vi "FPGA_Host_RealTime_Data_Viewer.vi"(3 "length":i32, 4 "Array":dbl[][](array[numeric]), 5 "Display Cluster":T1) -> ()   [LabVIEW 2023]
uses:
  TypeDefs/Display.ctl
  <vilib>/Analysis/baseanly.llb/Mean (DBL).vi
  User_Vi/Settings.vi
  <vilib>/Analysis/NI_AALBase.lvlib
panel:
  out "Current 3":bool=TRUE
  out "Forward Current3":dbl[][](array[numeric])
  out "Reverse Current3":dbl[][](array[numeric])
  out "Raster Current 3":dbl[][](array[numeric])
  out "Reverse Current2":dbl[][](array[numeric])
  out "Forward Current2":dbl[][](array[numeric])
  out "Current 2":bool=TRUE
  out "Raster Current 2":dbl[][](array[numeric])
  out "Current 1":bool=TRUE
  out "Reverse Current1":dbl[][](array[numeric])
  out "Forward Current1":dbl[][](array[numeric])
  out "Raster Current1":dbl[][](array[numeric])
  out "Raster Topo":dbl[][](array[numeric])
  out "Hop Current3":dbl[][](array[numeric])
  in  "Hop C3":bool=TRUE
  out "Hop Current2":dbl[][](array[numeric])
  in  "Hop C2":bool=TRUE
  out "Hop Current1":dbl[][](array[numeric])
  in  "Hop C1":bool=TRUE
  in  "Hop Top":bool=TRUE
  out "Hop Topography":dbl[][](array[numeric])
  out "Topology":bool=TRUE
  out "Reverse Topo":dbl[][](array[numeric])
  out "Forward Topo":dbl[][](array[numeric])
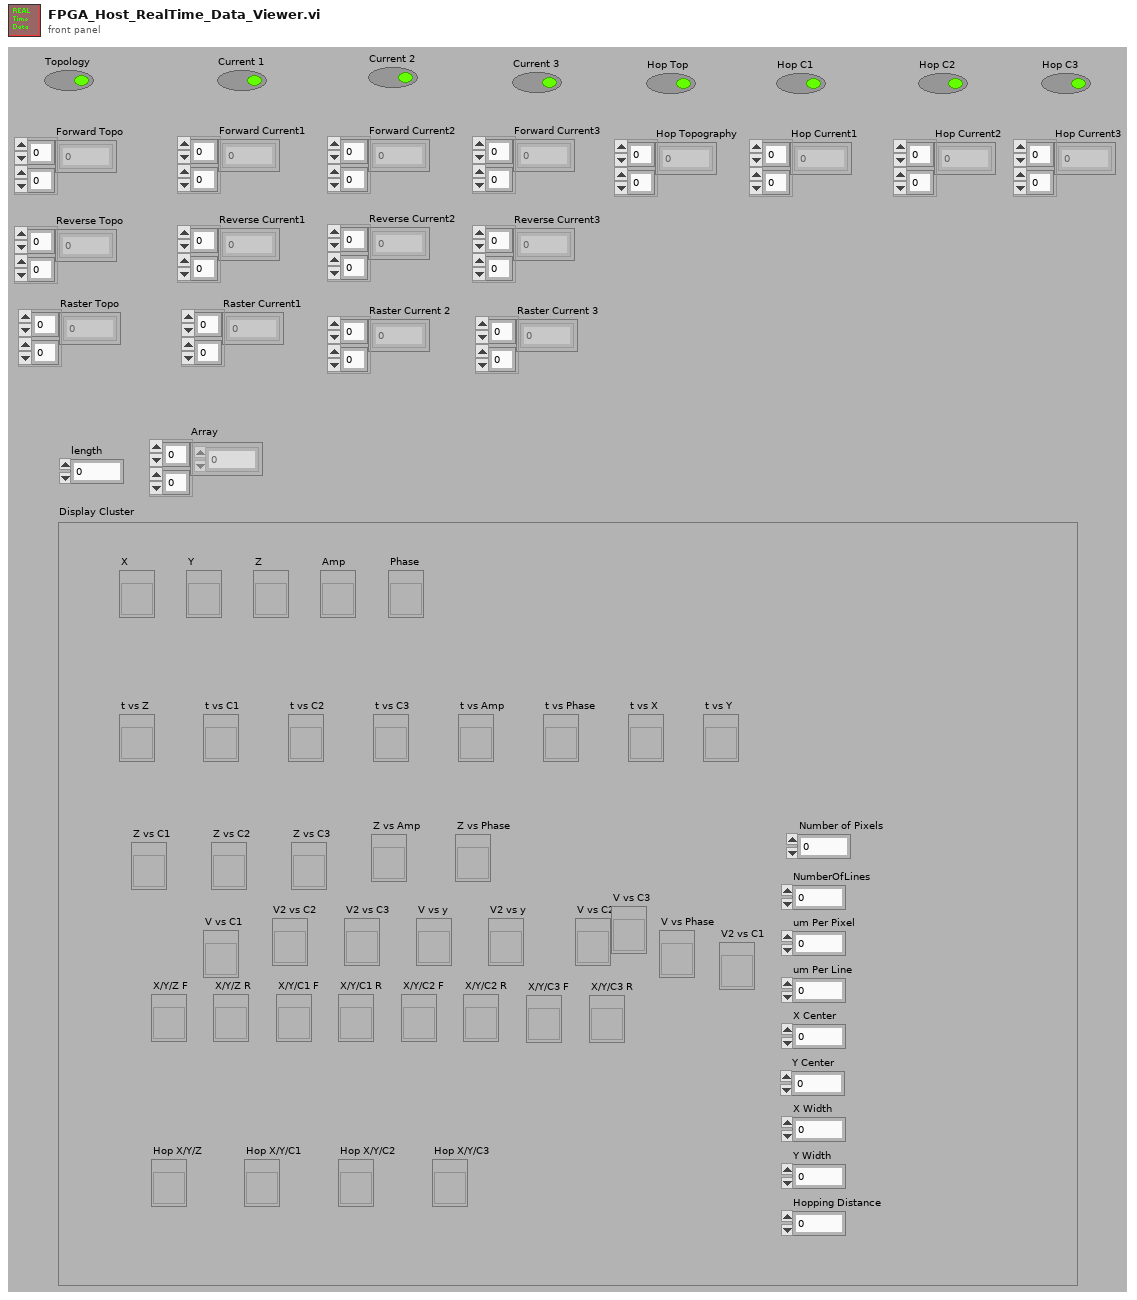
[diagram p1: front panel]
types:
  T1 = typedef "Display.ctl" = cluster{"X":refnum<vi>, "Y":refnum<vi>, "Z":refnum<vi>, "Amp":refnum<vi>, "Phase":refnum<vi>, "t vs Z":refnum<vi>, "t vs C1":refnum<vi>, "t vs C2":refnum<vi>, "t vs C3":refnum<vi>, "t vs Amp":refnum<vi>, "t vs Phase":refnum<vi>, "t vs X":refnum<vi>, "t vs Y":refnum<vi>, "Z vs C1":refnum<vi>, "Z vs C2":refnum<vi>, "Z vs C3":refnum<vi>, "V vs C1":refnum<vi>, "V vs C2":refnum<vi>, "V vs C3":refnum<vi>, "X/Y/Z F":refnum<vi>, "X/Y/Z R":refnum<vi>, "X/Y/C1 F":refnum<vi>, "X/Y/C1 R":refnum<vi>, "X/Y/C2 F":refnum<vi>, "X/Y/C2 R":refnum<vi>, "X/Y/C3 F":refnum<vi>, "X/Y/C3 R":refnum<vi>, "NumberOfLines":u16, "um Per Pixel":dbl, "um Per Line":dbl, "X Center":dbl, "Hop X/Y/Z":refnum<vi>, "Hop X/Y/C1":refnum<vi>, "Hop X/Y/C2":refnum<vi>, "Hop X/Y/C3":refnum<vi>, "X Width":dbl, "Y Width":dbl, "Hopping Distance":dbl, "V2 vs C1":refnum<vi>, "V vs Phase":refnum<vi>, "Y Center":dbl, "Number of Pixels":dbl, "V2 vs C2":refnum<vi>, "V2 vs C3":refnum<vi>, "V vs y":refnum<vi>, "V2 vs y":refnum<vi>, "Z vs Amp":refnum<vi>, "Z vs Phase":refnum<vi>}
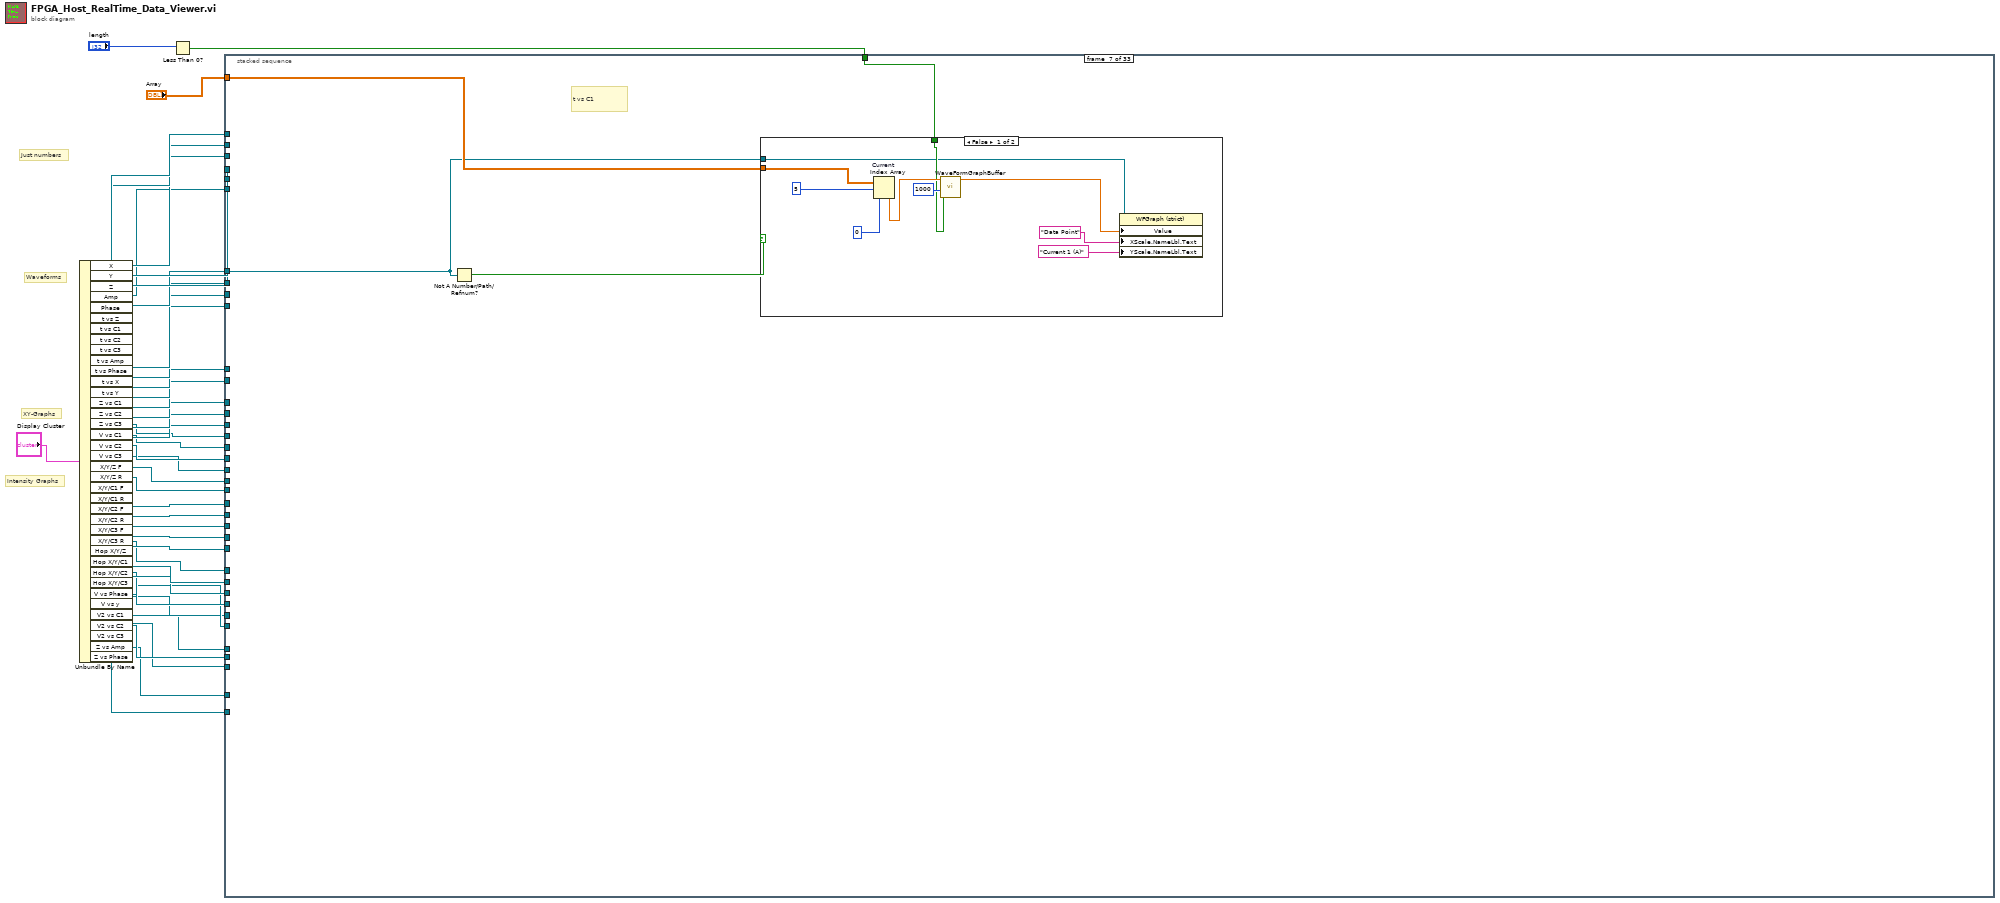
[diagram p0: block diagram]
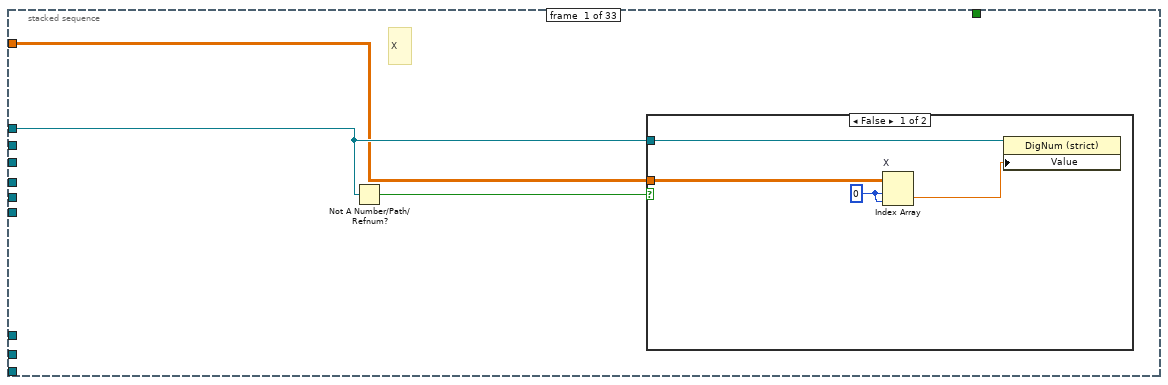
[diagram p2: hidden frame]
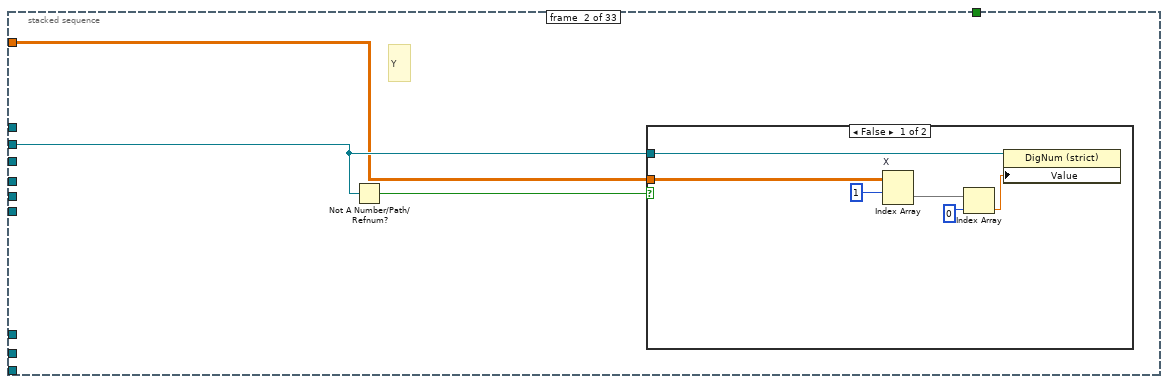
[diagram p4: hidden frame]
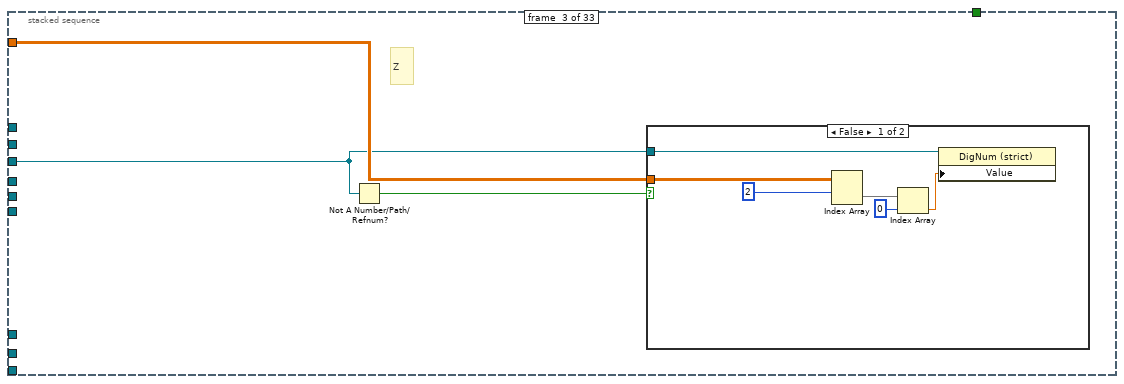
[diagram p6: hidden frame]
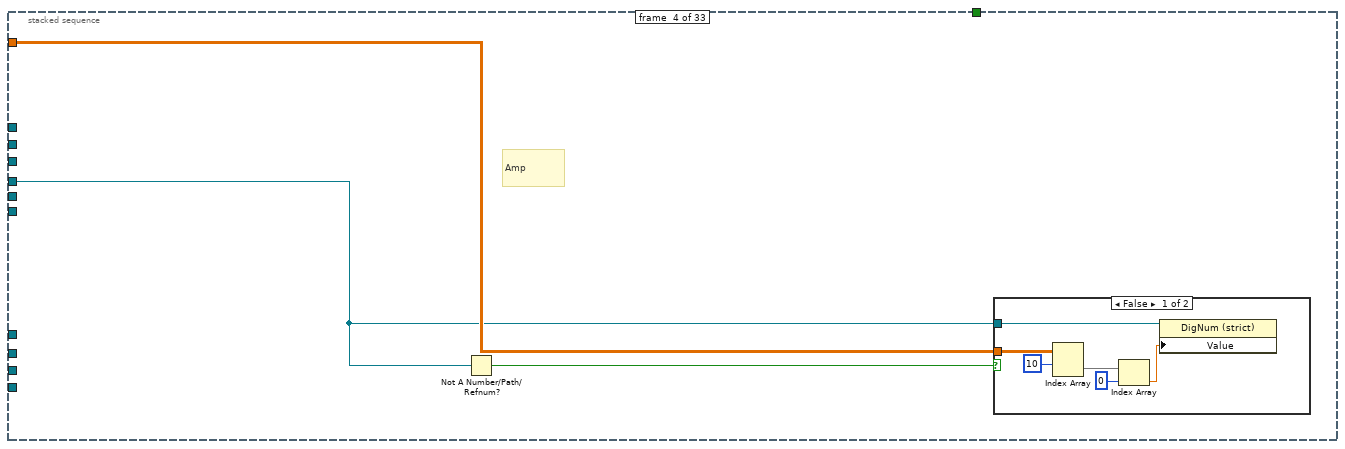
[diagram p8: hidden frame]
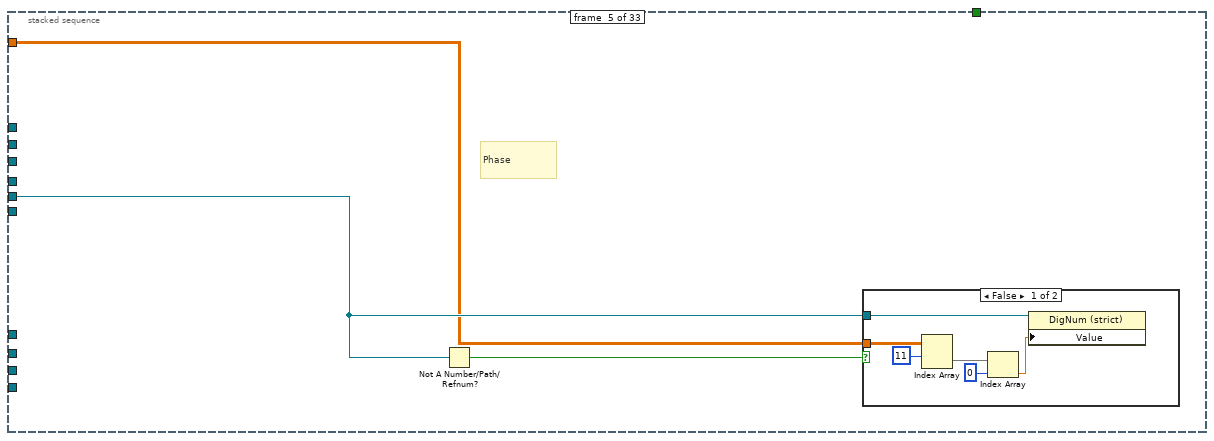
[diagram p10: hidden frame]
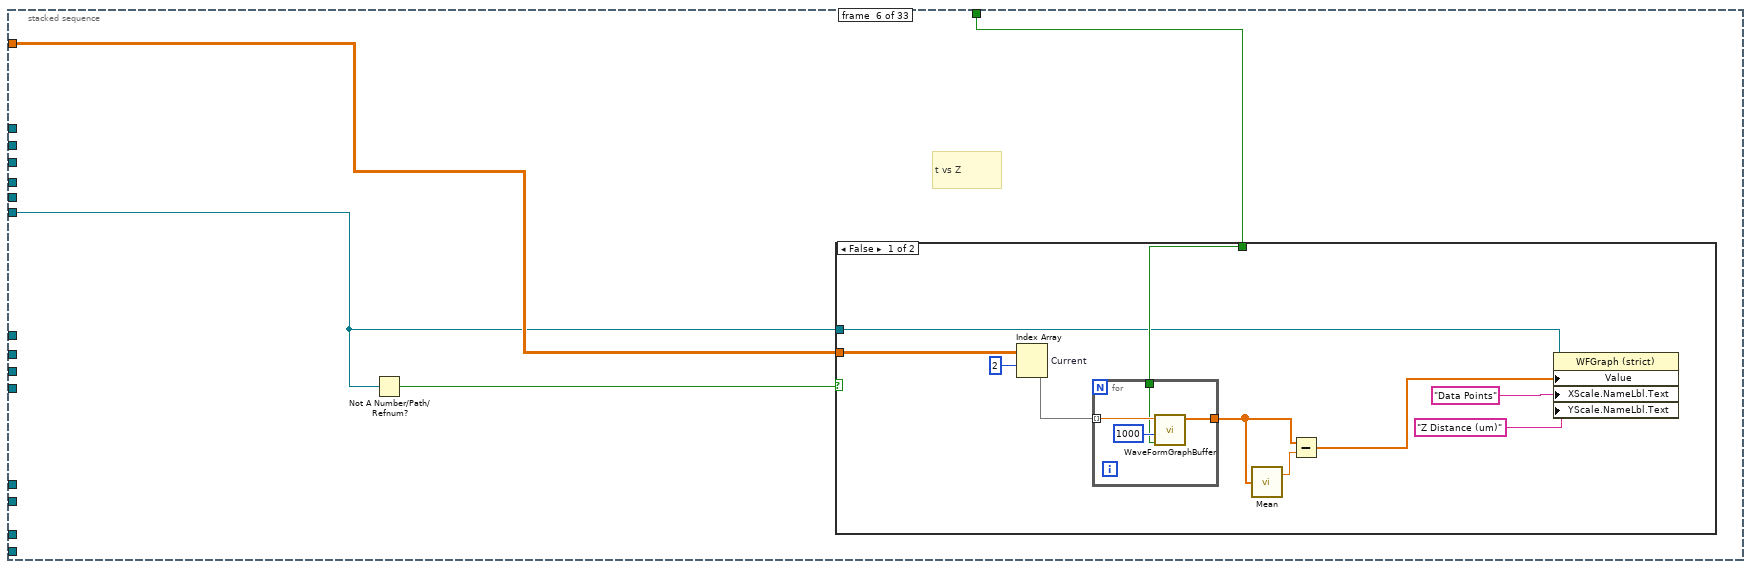
[diagram p12: hidden frame]
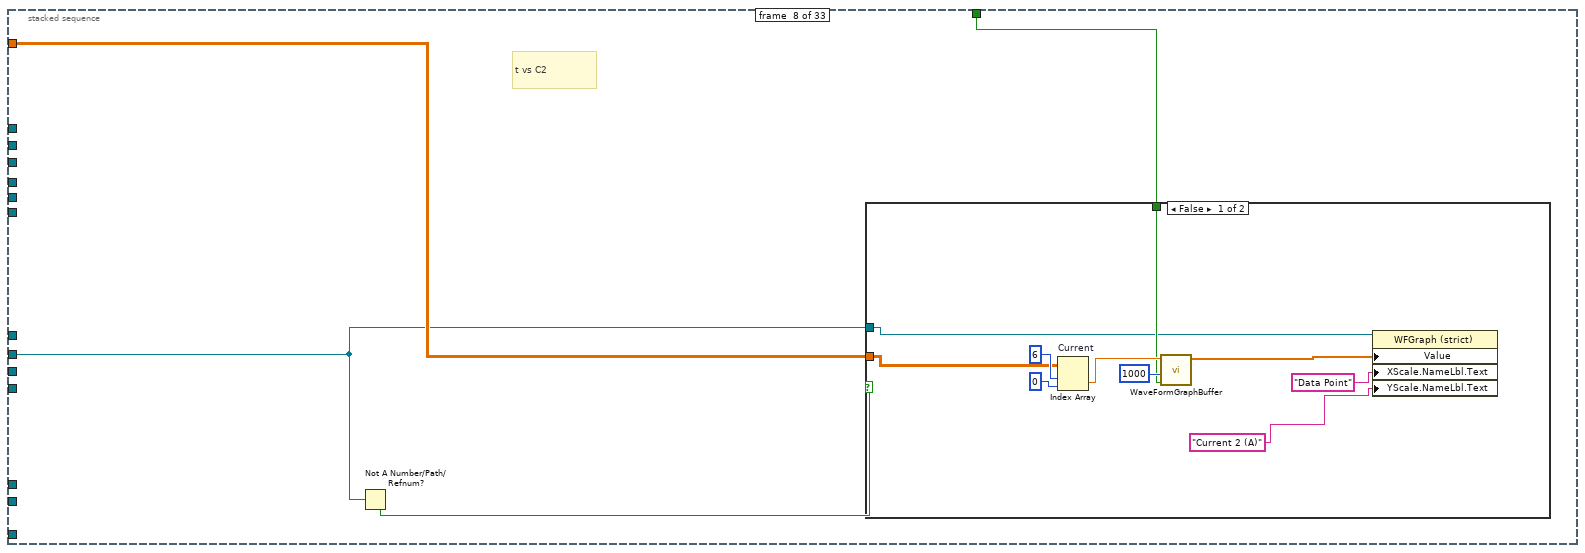
[diagram p15: hidden frame]
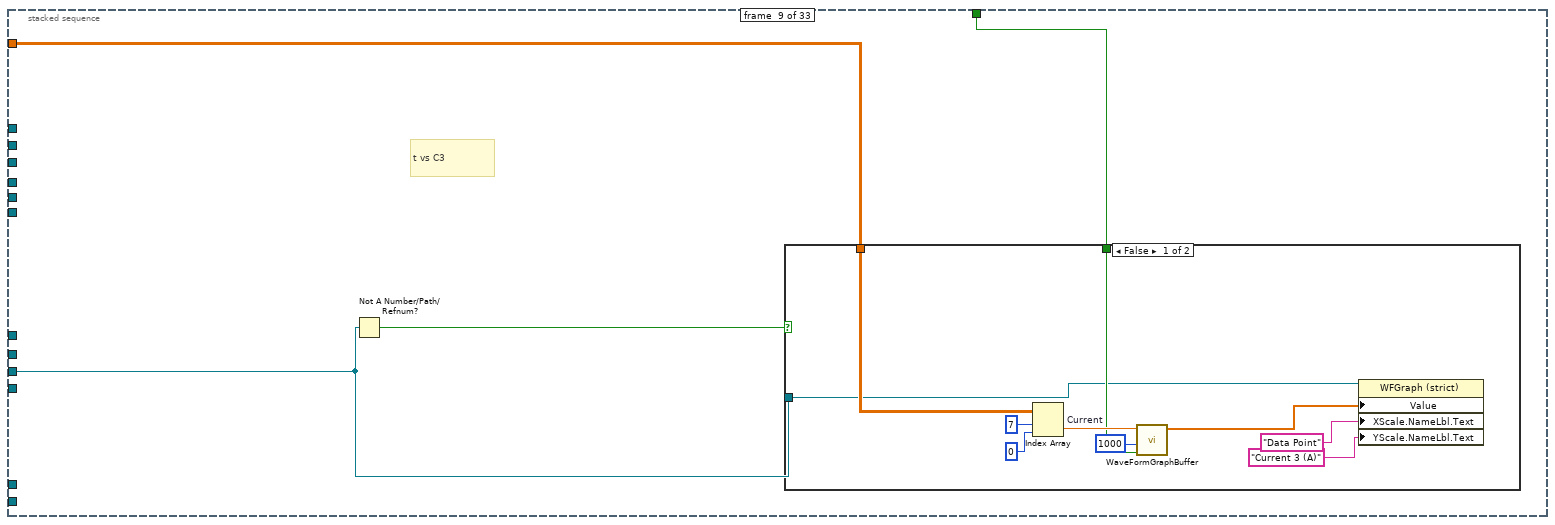
[diagram p17: hidden frame]
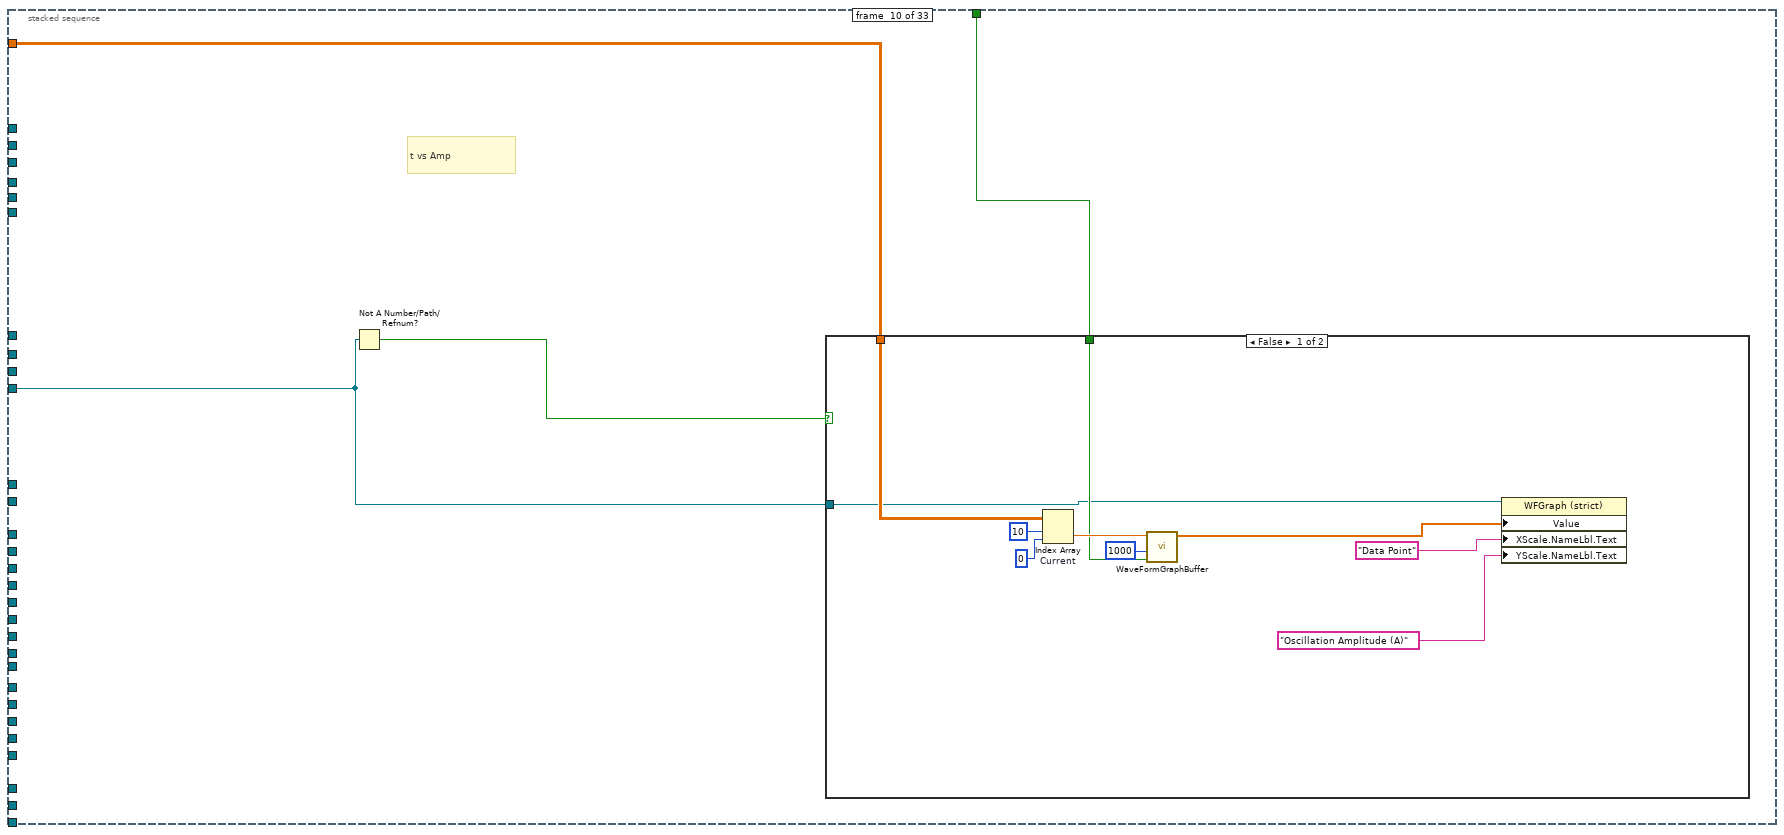
[diagram p19: hidden frame]
diagram:
  # "Intensity Graphs"
  # "XY-Graphs"
  # "Waveforms"
  # "Just numbers"
  n1 = Unbundle By Name("Display Cluster") -> ("X"=w38:refnum<vi>, "Y"=w37:refnum<vi>, "Z"=w36:refnum<vi>, "Amp"=w35:refnum<vi>, "Phase"=w34:refnum<vi>, "t vs Z"=w33:refnum<vi>, "t vs C1"=w32:refnum<vi>, "t vs C2"=w31:refnum<vi>, "t vs C3"=w30:refnum<vi>, "t vs Amp"=w29:refnum<vi>, "t vs Phase"=w28:refnum<vi>, "t vs X"=w27:refnum<vi>, "t vs Y"=w26:refnum<vi>, "Z vs C1"=w25:refnum<vi>, "Z vs C2"=w24:refnum<vi>, "Z vs C3"=w23:refnum<vi>, "V vs C1"=w22:refnum<vi>, "V vs C2"=w21:refnum<vi>, "V vs C3"=w20:refnum<vi>, "X/Y/Z F"=w19:refnum<vi>, "X/Y/Z R"=w18:refnum<vi>, "X/Y/C1 F"=w17:refnum<vi>, "X/Y/C1 R"=w16:refnum<vi>, "X/Y/C2 F"=w15:refnum<vi>, "X/Y/C2 R"=w14:refnum<vi>, "X/Y/C3 F"=w13:refnum<vi>, "X/Y/C3 R"=w6:refnum<vi>, "Hop X/Y/Z"=w12:refnum<vi>, "Hop X/Y/C1"=w11:refnum<vi>, "Hop X/Y/C2"=w10:refnum<vi>, "Hop X/Y/C3"=w7:refnum<vi>, "V vs Phase"=w8:refnum<vi>, "V2 vs C1"=w4:refnum<vi>, "V2 vs C2"=w5:refnum<vi>, "V2 vs C3"=w3:refnum<vi>, "Z vs Amp"=w2:refnum<vi>, "Z vs Phase"=w1:refnum<vi>)  [unwired: 1 out]
  n2 = Less Than 0?(x="length") -> (x < 0?=w40:bool)
  n3 = stacked-sequence {
    tunnel: w38 -> [w43 _ _ _ _ _ _ _ _ _ _ _ _ _ _ _ _ _ _ _ _ _ _ _ _ _ _ _ _ _ _ _ _]
    tunnel: w37 -> [_ w50 _ _ _ _ _ _ _ _ _ _ _ _ _ _ _ _ _ _ _ _ _ _ _ _ _ _ _ _ _ _ _]
    tunnel: w36 -> [_ _ w58 _ _ _ _ _ _ _ _ _ _ _ _ _ _ _ _ _ _ _ _ _ _ _ _ _ _ _ _ _ _]
    tunnel: w32 -> [_ _ _ _ _ _ w103 _ _ _ _ _ _ _ _ _ _ _ _ _ _ _ _ _ _ _ _ _ _ _ _ _ _]
    tunnel: w31 -> [_ _ _ _ _ _ _ w117 _ _ _ _ _ _ _ _ _ _ _ _ _ _ _ _ _ _ _ _ _ _ _ _ _]
    tunnel: w30 -> [_ _ _ _ _ _ _ _ w131 _ _ _ _ _ _ _ _ _ _ _ _ _ _ _ _ _ _ _ _ _ _ _ _]
    tunnel: w29 -> [_ _ _ _ _ _ _ _ _ w145 _ _ _ _ _ _ _ _ _ _ _ _ _ _ _ _ _ _ _ _ _ _ _]
    tunnel: w28 -> [_ _ _ _ _ _ _ _ _ _ w159 _ _ _ _ _ _ _ _ _ _ _ _ _ _ _ _ _ _ _ _ _ _]
    tunnel: w25 -> [_ _ _ _ _ _ _ _ _ _ _ _ _ w203 _ _ _ _ _ _ _ _ _ _ _ _ _ _ _ _ _ _ _]
    tunnel: w24 -> [_ _ _ _ _ _ _ _ _ _ _ _ _ _ _ _ w266 _ _ _ _ _ _ _ _ _ _ _ _ _ _ _ _]
    tunnel: w23 -> [_ _ _ _ _ _ _ _ _ _ _ _ _ _ _ _ _ w285 _ _ _ _ _ _ _ _ _ _ _ _ _ _ _]
    tunnel: w22 -> [_ _ _ _ _ _ _ _ _ _ _ _ _ _ _ _ _ _ w308 _ _ _ _ _ _ _ _ _ _ _ _ _ _]
    tunnel: w21 -> [_ _ _ _ _ _ _ _ _ _ _ _ _ _ _ _ _ _ _ w327 _ _ _ _ _ _ _ _ _ _ _ _ _]
    tunnel: w20 -> [_ _ _ _ _ _ _ _ _ _ _ _ _ _ _ _ _ _ _ _ w349 _ _ _ _ _ _ _ _ _ _ _ _]
    tunnel: "Array" -> [w42 w49 w59 w68 w76 w87 w105 w119 w132 w146 w160 w174 w188 w201 w223 w244 w265 w286 w307 w329 w348 w371 w515 w657 w799 w939 w1066 w1193 w1320 w1445 w1466 w1487 w1508]
    tunnel: w40 -> [_ _ _ _ _ w85 w104 w118 w133 w147 w161 w173 w187 w202 w224 w245 w264 w287 w306 w328 w350 _ _ _ _ _ _ _ _ w1446 w1467 w1488 w1509]
    tunnel: w35 -> [_ _ _ w67 _ _ _ _ _ _ _ _ _ _ _ _ _ _ _ _ _ _ _ _ _ _ _ _ _ _ _ _ _]
    tunnel: w34 -> [_ _ _ _ w77 _ _ _ _ _ _ _ _ _ _ _ _ _ _ _ _ _ _ _ _ _ _ _ _ _ _ _ _]
    tunnel: w33 -> [_ _ _ _ _ w86 _ _ _ _ _ _ _ _ _ _ _ _ _ _ _ _ _ _ _ _ _ _ _ _ _ _ _]
    tunnel: w27 -> [_ _ _ _ _ _ _ _ _ _ _ w175 _ _ _ _ _ _ _ _ _ _ _ _ _ _ _ _ _ _ _ _ _]
    tunnel: w19 -> [_ _ _ _ _ _ _ _ _ _ _ _ _ _ _ _ _ _ _ _ _ w376 _ _ _ _ _ _ _ _ _ _ _]
    tunnel: w18 -> [_ _ _ _ _ _ _ _ _ _ _ _ _ _ _ _ _ _ _ _ _ w375 _ _ _ _ _ _ _ _ _ _ _]
    tunnel: w17 -> [_ _ _ _ _ _ _ _ _ _ _ _ _ _ _ _ _ _ _ _ _ _ w514 _ _ _ _ _ _ _ _ _ _]
    tunnel: w16 -> [_ _ _ _ _ _ _ _ _ _ _ _ _ _ _ _ _ _ _ _ _ _ w513 _ _ _ _ _ _ _ _ _ _]
    tunnel: w15 -> [_ _ _ _ _ _ _ _ _ _ _ _ _ _ _ _ _ _ _ _ _ _ _ w656 _ _ _ _ _ _ _ _ _]
    tunnel: w14 -> [_ _ _ _ _ _ _ _ _ _ _ _ _ _ _ _ _ _ _ _ _ _ _ w655 _ _ _ _ _ _ _ _ _]
    tunnel: w13 -> [_ _ _ _ _ _ _ _ _ _ _ _ _ _ _ _ _ _ _ _ _ _ _ _ w798 _ _ _ _ _ _ _ _]
    tunnel: w6 -> [_ _ _ _ _ _ _ _ _ _ _ _ _ _ _ _ _ _ _ _ _ _ _ _ w797 _ _ _ _ _ _ _ _]
    tunnel: w26 -> [_ _ _ _ _ _ _ _ _ _ _ _ w189 _ _ _ _ _ _ _ _ _ _ _ _ _ _ _ _ _ _ _ _]
    tunnel: w12 -> [_ _ _ _ _ _ _ _ _ _ _ _ _ _ _ _ _ _ _ _ _ _ _ _ _ w938 _ _ _ _ _ _ _]
    tunnel: w11 -> [_ _ _ _ _ _ _ _ _ _ _ _ _ _ _ _ _ _ _ _ _ _ _ _ _ _ w1064 _ _ _ _ _ _]
    tunnel: w10 -> [_ _ _ _ _ _ _ _ _ _ _ _ _ _ _ _ _ _ _ _ _ _ _ _ _ _ _ w1191 _ _ _ _ _]
    tunnel: w7 -> [_ _ _ _ _ _ _ _ _ _ _ _ _ _ _ _ _ _ _ _ _ _ _ _ _ _ _ _ w1318 _ _ _ _]
    tunnel: w8 -> [_ _ _ _ _ _ _ _ _ _ _ _ _ _ _ _ _ _ _ _ _ _ _ _ _ _ _ _ _ w1447 _ _ _]
    tunnel: w5 -> [_ _ _ _ _ _ _ _ _ _ _ _ _ _ _ _ _ _ _ _ _ _ _ _ _ _ _ _ _ _ _ w1486 _]
    tunnel: w4 -> [_ _ _ _ _ _ _ _ _ _ _ _ _ _ _ _ _ _ _ _ _ _ _ _ _ _ _ _ _ _ w1465 _ _]
    tunnel: w3 -> [_ _ _ _ _ _ _ _ _ _ _ _ _ _ _ _ _ _ _ _ _ _ _ _ _ _ _ _ _ _ _ _ w1507]
    tunnel: w2 -> [_ _ _ _ _ _ _ _ _ _ _ _ _ _ w222 _ _ _ _ _ _ _ _ _ _ _ _ _ _ _ _ _ _]
    tunnel: w1 -> [_ _ _ _ _ _ _ _ _ _ _ _ _ _ _ w243 _ _ _ _ _ _ _ _ _ _ _ _ _ _ _ _ _]
    frame #0 {
      # "X"
      n4 = Not A Number/Path/Refnum?(number/path/refnum=w43) -> (NaN/Path/Refnum?=w44:bool)
      n5 = case shown="False" w44 {
        tunnel: w43 -> [w48 _]
        tunnel: w42 -> [w47 _]
        frame False {
          w46 = 0 ("index (row)")
          n6 = Index Array "X"(array=w47, index (row)=w46, index (col)=w46) -> (element=w45:dbl)
          n7 = property class="DigNum (strict)"(reference=w48, "Value"=w45) -> ()  [unwired: 1 in, 2 out]
        }
        frame True {
        }
      }
    }
    frame #1 {
      # "Y"
      n8 = Not A Number/Path/Refnum?(number/path/refnum=w50) -> (NaN/Path/Refnum?=w51:bool)
      n9 = case shown="False" w51 {
        tunnel: w50 -> [w53 _]
        tunnel: w49 -> [w52 _]
        frame False {
          n10 = Index Array "X"(array=w52, index (row)=1) -> (element=w56:dbl[])  [unwired: 1 in]
          n11 = Index Array(array=w56, index=0) -> (element=w57:dbl)
          n12 = property class="DigNum (strict)"(reference=w53, "Value"=w57) -> ()  [unwired: 1 in, 2 out]
        }
        frame True {
        }
      }
    }
    frame #2 {
      # "Z"
      n13 = Not A Number/Path/Refnum?(number/path/refnum=w58) -> (NaN/Path/Refnum?=w60:bool)
      n14 = case shown="False" w60 {
        tunnel: w59 -> [w62 _]
        tunnel: w58 -> [w61 _]
        frame False {
          n15 = Index Array(array=w62, index (row)=2) -> (element=w64:dbl[])  [unwired: 1 in]
          n16 = Index Array(array=w64, index=0) -> (element=w63:dbl)
          n17 = property class="DigNum (strict)"(reference=w61, "Value"=w63) -> ()  [unwired: 1 in, 2 out]
        }
        frame True {
        }
      }
    }
    frame #3 {
      # "Amp"
      n18 = Not A Number/Path/Refnum?(number/path/refnum=w67) -> (NaN/Path/Refnum?=w69:bool)
      n19 = case shown="False" w69 {
        tunnel: w68 -> [w71 _]
        tunnel: w67 -> [w70 _]
        frame False {
          n20 = Index Array(array=w71, index (row)=10) -> (element=w73:dbl[])  [unwired: 1 in]
          n21 = Index Array(array=w73, index=0) -> (element=w72:dbl)
          n22 = property class="DigNum (strict)"(reference=w70, "Value"=w72) -> ()  [unwired: 1 in, 2 out]
        }
        frame True {
        }
      }
    }
    frame #4 {
      # "Phase"
      n23 = Not A Number/Path/Refnum?(number/path/refnum=w77) -> (NaN/Path/Refnum?=w78:bool)
      n24 = case shown="False" w78 {
        tunnel: w76 -> [w80 _]
        tunnel: w77 -> [w79 _]
        frame False {
          n25 = Index Array(array=w80, index (row)=11) -> (element=w82:dbl[])  [unwired: 1 in]
          n26 = Index Array(array=w82, index=0) -> (element=w81:dbl)
          n27 = property class="DigNum (strict)"(reference=w79, "Value"=w81) -> ()  [unwired: 1 in, 2 out]
        }
        frame True {
        }
      }
    }
    frame #5 {
      # "t vs Z"
      n28 = Not A Number/Path/Refnum?(number/path/refnum=w86) -> (NaN/Path/Refnum?=w88:bool)
      n29 = case shown="False" w88 {
        tunnel: w87 -> [w96 _]
        tunnel: w85 -> [w95 _]
        tunnel: w86 -> [w94 _]
        frame False {
          n30 = Index Array "Current"(array=w96, index (row)=2) -> (element=w97:dbl[])  [unwired: 1 in]
          n31 = for {
            tunnel: [w101] -> w90
            tunnel: w97 -> [w100] mode=indexing
            tunnel: w95 -> [w99]
            n32 = call "WaveFormGraphBuffer.vi"("clear first (no:F)"=w99, "chart length (points)"=1000, "NewPoint"=w100) -> ("Value"=w101:dbl[])  [unwired: 8 in]
          }
          n33 = call-poly <vilib>:"Mean.vi"("X"=w90) -> ("mean"=w91:dbl)  [unwired: 1 out]
          n34 = Subtract(x=w90, y=w91) -> (x-y=w89:dbl[])
          n35 = property class="WFGraph (strict)"(reference=w94, "Value"=w89, "XScale.NameLbl.Text"="Data Points" ("X Scale.Name Label.Text"), "YScale.NameLbl.Text"="Z Distance (um)" ("Y Scale.Name Label.Text")) -> ()  [unwired: 1 in, 2 out]
        }
        frame True {
        }
      }
    }
    frame #6 {
      # "t vs C1"
      n36 = Not A Number/Path/Refnum?(number/path/refnum=w103) -> (NaN/Path/Refnum?=w106:bool)
      n37 = case shown="False" w106 {
        tunnel: w105 -> [w111 _]
        tunnel: w104 -> [w110 _]
        tunnel: w103 -> [w109 _]
        frame False {
          n38 = Index Array "Current"(array=w111, index (row)=5, index (col)=0 ("disabled index (col)")) -> (element=w112:dbl)
          n39 = call "WaveFormGraphBuffer.vi"("clear first (no:F)"=w110, "chart length (points)"=1000, "NewPoint"=w112) -> ("Value"=w113:dbl[])  [unwired: 8 in]
          n40 = property class="WFGraph (strict)"(reference=w109, "Value"=w113, "XScale.NameLbl.Text"="Data Point" ("X Scale.Name Label.Text"), "YScale.NameLbl.Text"="Current 1 (A)" ("Y Scale.Name Label.Text")) -> ()  [unwired: 1 in, 2 out]
        }
        frame True {
        }
      }
    }
    frame #7 {
      # "t vs C2"
      n41 = Not A Number/Path/Refnum?(number/path/refnum=w117) -> (NaN/Path/Refnum?=w120:bool)
      n42 = case shown="False" w120 {
        tunnel: w119 -> [w125 _]
        tunnel: w118 -> [w124 _]
        tunnel: w117 -> [w123 _]
        frame False {
          n43 = Index Array "Current"(array=w125, index (row)=6, index (col)=0 ("disabled index (col)")) -> (element=w130:dbl)
          n44 = call "WaveFormGraphBuffer.vi"("clear first (no:F)"=w124, "chart length (points)"=1000, "NewPoint"=w130) -> ("Value"=w129:dbl[])  [unwired: 8 in]
          n45 = property class="WFGraph (strict)"(reference=w123, "Value"=w129, "XScale.NameLbl.Text"="Data Point" ("X Scale.Name Label.Text"), "YScale.NameLbl.Text"="Current 2 (A)" ("Y Scale.Name Label.Text")) -> ()  [unwired: 1 in, 2 out]
        }
        frame True {
        }
      }
    }
    frame #8 {
      # "t vs C3"
      n46 = Not A Number/Path/Refnum?(number/path/refnum=w131) -> (NaN/Path/Refnum?=w134:bool)
      n47 = case shown="False" w134 {
        tunnel: w133 -> [w139 _]
        tunnel: w132 -> [w138 _]
        tunnel: w131 -> [w137 _]
        frame False {
          n48 = Index Array "Current"(array=w138, index (row)=7, index (col)=0 ("disabled index (col)")) -> (element=w144:dbl)
          n49 = call "WaveFormGraphBuffer.vi"("clear first (no:F)"=w139, "chart length (points)"=1000, "NewPoint"=w144) -> ("Value"=w143:dbl[])  [unwired: 8 in]
          n50 = property class="WFGraph (strict)"(reference=w137, "Value"=w143, "XScale.NameLbl.Text"="Data Point" ("X Scale.Name Label.Text"), "YScale.NameLbl.Text"="Current 3 (A)" ("Y Scale.Name Label.Text")) -> ()  [unwired: 1 in, 2 out]
        }
        frame True {
        }
      }
    }
    frame #9 {
      # "t vs Amp"
      n51 = Not A Number/Path/Refnum?(number/path/refnum=w145) -> (NaN/Path/Refnum?=w148:bool)
      n52 = case shown="False" w148 {
        tunnel: w147 -> [w153 _]
        tunnel: w146 -> [w152 _]
        tunnel: w145 -> [w151 _]
        frame False {
          n53 = Index Array "Current"(array=w152, index (row)=10, index (col)=0 ("disabled index (col)")) -> (element=w158:dbl)
          n54 = call "WaveFormGraphBuffer.vi"("clear first (no:F)"=w153, "chart length (points)"=1000, "NewPoint"=w158) -> ("Value"=w157:dbl[])  [unwired: 8 in]
          n55 = property class="WFGraph (strict)"(reference=w151, "Value"=w157, "XScale.NameLbl.Text"="Data Point" ("X Scale.Name Label.Text"), "YScale.NameLbl.Text"="Oscillation Amplitude (A)" ("Y Scale.Name Label.Text")) -> ()  [unwired: 1 in, 2 out]
        }
        frame True {
        }
      }
    }
    frame #10 {
      # "t vs Phase"
      n56 = Not A Number/Path/Refnum?(number/path/refnum=w159) -> (NaN/Path/Refnum?=w162:bool)
      n57 = case shown="False" w162 {
        tunnel: w161 -> [w167 _]
        tunnel: w160 -> [w166 _]
        tunnel: w159 -> [w165 _]
        frame False {
          n58 = Index Array "Current"(array=w166, index (row)=11, index (col)=0 ("disabled index (col)")) -> (element=w172:dbl)
          n59 = call "WaveFormGraphBuffer.vi"("clear first (no:F)"=w167, "chart length (points)"=1000, "NewPoint"=w172) -> ("Value"=w171:dbl[])  [unwired: 8 in]
          n60 = property class="WFGraph (strict)"(reference=w165, "Value"=w171, "XScale.NameLbl.Text"="Data Point" ("X Scale.Name Label.Text"), "YScale.NameLbl.Text"="Oscillation Phase" ("Y Scale.Name Label.Text")) -> ()  [unwired: 1 in, 2 out]
        }
        frame True {
        }
      }
    }
    frame #11 {
      # "t vs X"
      n61 = Not A Number/Path/Refnum?(number/path/refnum=w175) -> (NaN/Path/Refnum?=w176:bool)
      n62 = case shown="False" w176 {
        tunnel: w173 -> [w181 _]
        tunnel: w174 -> [w180 _]
        tunnel: w175 -> [w179 _]
        frame False {
          n63 = Index Array "Current"(array=w180, index (row)=0, index (col)=0 ("disabled index (col)")) -> (element=w186:dbl)
          n64 = call "WaveFormGraphBuffer.vi"("clear first (no:F)"=w181, "chart length (points)"=1000, "NewPoint"=w186) -> ("Value"=w185:dbl[])  [unwired: 8 in]
          n65 = property class="WFGraph (strict)"(reference=w179, "Value"=w185, "XScale.NameLbl.Text"="Data Point" ("X Scale.Name Label.Text"), "YScale.NameLbl.Text"="X Position (um)" ("Y Scale.Name Label.Text")) -> ()  [unwired: 1 in, 2 out]
        }
        frame True {
        }
      }
    }
    frame #12 {
      # "t vs Y"
      n66 = Not A Number/Path/Refnum?(number/path/refnum=w189) -> (NaN/Path/Refnum?=w190:bool)
      n67 = case shown="False" w190 {
        tunnel: w187 -> [w195 _]
        tunnel: w188 -> [w194 _]
        tunnel: w189 -> [w193 _]
        frame False {
          n68 = Index Array "Current"(array=w194, index (row)=1, index (col)=0 ("disabled index (col)")) -> (element=w200:dbl)
          n69 = call "WaveFormGraphBuffer.vi"("clear first (no:F)"=w195, "chart length (points)"=1000, "NewPoint"=w200) -> ("Value"=w199:dbl[])  [unwired: 8 in]
          n70 = property class="WFGraph (strict)"(reference=w193, "Value"=w199, "XScale.NameLbl.Text"="Data Point" ("X Scale.Name Label.Text"), "YScale.NameLbl.Text"="Y Postion (um)" ("Y Scale.Name Label.Text")) -> ()  [unwired: 1 in, 2 out]
        }
        frame True {
        }
      }
    }
    frame #13 {
      # "Z vs C1"
      n71 = Not A Number/Path/Refnum?(number/path/refnum=w203) -> (NaN/Path/Refnum?=w204:bool)
      n72 = case shown="False" w204 {
        tunnel: w203 -> [w213 _]
        tunnel: w202 -> [w212 _]
        tunnel: w201 -> [w211 _]
        frame False {
          n73 = Index Array ("Oscillation Amplitude")(array=w211, index (row)=2 ("disabled index (row)"), index (col)=0) -> (element=w210:dbl)
          n74 = Index Array ("Oscillation Amplitude")(array=w211, index (row)=5 ("disabled index (row)"), index (col)=0) -> (element=w208:dbl)
          n75 = call "XY Chart Buffer_PINK.vi"("clear first (no:F)"=w212, "chart length (points)"=10000, "YNew"=w208, "XNew"=w210) -> ("Value Y"=w221:dbl[], "Value X"=w220:dbl[])  [unwired: 6 in]
          n76 = Bundle("Value X"=w220, "Value Y"=w221) -> (w219:cluster{"Value X":dbl[], "Value Y":dbl[]})  [unwired: 1 in]
          n77 = Build Array(w219) -> (w214:cluster{"Value X":dbl[], "Value Y":dbl[]}[])
          n78 = property class="XYGraph (strict)"(reference=w213, "Value"=w214, "XScale.NameLbl.Text"="Z Distance (um)" ("X Scale.Name Label.Text"), "YScale.NameLbl.Text"="Current 1 (nA)" ("Y Scale.Name Label.Text"), "YScale.Multiplier"=1000000000.0 ("Y Scale.Offset and Multiplier:Multiplier")) -> ()  [unwired: 1 in, 2 out]
        }
        frame True {
        }
      }
    }
    frame #14 {
      # "Z vs Amp"
      n79 = Not A Number/Path/Refnum?(number/path/refnum=w222) -> (NaN/Path/Refnum?=w225:bool)
      n80 = case shown="False" w225 {
        tunnel: w222 -> [w234 _]
        tunnel: w224 -> [w233 _]
        tunnel: w223 -> [w232 _]
        frame False {
          n81 = Index Array ("Oscillation Amplitude")(array=w232, index (row)=2 ("disabled index (row)"), index (col)=0) -> (element=w231:dbl)
          n82 = Index Array ("Oscillation Amplitude")(array=w232, index (row)=10 ("disabled index (row)"), index (col)=0) -> (element=w229:dbl)
          n83 = call "XY Chart Buffer_PINK.vi"("clear first (no:F)"=w233, "chart length (points)"=10000, "YNew"=w229, "XNew"=w231) -> ("Value Y"=w242:dbl[], "Value X"=w241:dbl[])  [unwired: 6 in]
          n84 = Bundle("Value X"=w241, "Value Y"=w242) -> (w240:cluster{"Value X":dbl[], "Value Y":dbl[]})  [unwired: 1 in]
          n85 = Build Array(w240) -> (w235:cluster{"Value X":dbl[], "Value Y":dbl[]}[])
          n86 = property class="XYGraph (strict)"(reference=w234, "Value"=w235, "XScale.NameLbl.Text"="Z Distance (um)" ("X Scale.Name Label.Text"), "YScale.NameLbl.Text"="Amplitude (nA)" ("Y Scale.Name Label.Text"), "YScale.Multiplier"=1000000000.0 ("Y Scale.Offset and Multiplier:Multiplier")) -> ()  [unwired: 1 in, 2 out]
        }
        frame True {
        }
      }
    }
    frame #15 {
      # "Z vs Phase"
      n87 = Not A Number/Path/Refnum?(number/path/refnum=w243) -> (NaN/Path/Refnum?=w246:bool)
      n88 = case shown="False" w246 {
        tunnel: w243 -> [w255 _]
        tunnel: w245 -> [w254 _]
        tunnel: w244 -> [w253 _]
        frame False {
          n89 = Index Array ("Oscillation Amplitude")(array=w253, index (row)=2 ("disabled index (row)"), index (col)=0) -> (element=w252:dbl)
          n90 = Index Array ("Oscillation Amplitude")(array=w253, index (row)=11 ("disabled index (row)"), index (col)=0) -> (element=w250:dbl)
          n91 = call "XY Chart Buffer_PINK.vi"("clear first (no:F)"=w254, "chart length (points)"=10000, "YNew"=w250, "XNew"=w252) -> ("Value Y"=w263:dbl[], "Value X"=w262:dbl[])  [unwired: 6 in]
          n92 = Bundle("Value X"=w262, "Value Y"=w263) -> (w261:cluster{"Value X":dbl[], "Value Y":dbl[]})  [unwired: 1 in]
          n93 = Build Array(w261) -> (w256:cluster{"Value X":dbl[], "Value Y":dbl[]}[])
          n94 = property class="XYGraph (strict)"(reference=w255, "Value"=w256, "XScale.NameLbl.Text"="Z Distance (um)" ("X Scale.Name Label.Text"), "YScale.NameLbl.Text"="Phase" ("Y Scale.Name Label.Text"), "YScale.Multiplier"=1.0 ("Y Scale.Offset and Multiplier:Multiplier")) -> ()  [unwired: 1 in, 2 out]
        }
        frame True {
        }
      }
    }
    frame #16 {
      # "Z vs C2"
      n95 = Not A Number/Path/Refnum?(number/path/refnum=w266) -> (NaN/Path/Refnum?=w267:bool)
      n96 = case shown="False" w267 {
        tunnel: w266 -> [w273 _]
        tunnel: w265 -> [w271 _]
        tunnel: w264 -> [w272 _]
        frame False {
          n97 = Index Array ("Oscillation Amplitude")(array=w271, index (row)=2 ("disabled index (row)"), index (col)=0) -> (element=w276:dbl)
          n98 = Index Array ("Oscillation Amplitude")(array=w271, index (row)=6 ("disabled index (row)"), index (col)=0) -> (element=w274:dbl)
          n99 = call "XY Chart Buffer_PINK.vi"("clear first (no:F)"=w272, "chart length (points)"=10000, "YNew"=w274, "XNew"=w276) -> ("Value Y"=w284:dbl[], "Value X"=w283:dbl[])  [unwired: 6 in]
          n100 = Bundle("Value X"=w283, "Value Y"=w284) -> (w282:cluster{"Value X":dbl[], "Value Y":dbl[]})  [unwired: 1 in]
          n101 = Build Array(w282) -> (w277:cluster{"Value X":dbl[], "Value Y":dbl[]}[])
          n102 = property class="XYGraph (strict)"(reference=w273, "Value"=w277, "XScale.NameLbl.Text"="Z Distance (um)" ("X Scale.Name Label.Text"), "YScale.NameLbl.Text"="Current 2 (nA)" ("Y Scale.Name Label.Text"), "YScale.Multiplier"=1000000000.0 ("Y Scale.Offset and Multiplier:Multiplier")) -> ()  [unwired: 1 in, 2 out]
        }
        frame True {
        }
      }
    }
    frame #17 {
      # "Z vs C3"
      n103 = Not A Number/Path/Refnum?(number/path/refnum=w285) -> (NaN/Path/Refnum?=w288:bool)
      n104 = case shown="False" w288 {
        tunnel: w287 -> [w294 _]
        tunnel: w286 -> [w293 _]
        tunnel: w285 -> [w292 _]
        frame False {
          n105 = Index Array ("Oscillation Amplitude")(array=w293, index (row)=2 ("disabled index (row)"), index (col)=0) -> (element=w297:dbl)
          n106 = Index Array ("Oscillation Amplitude")(array=w293, index (row)=7 ("disabled index (row)"), index (col)=0) -> (element=w295:dbl)
          n107 = call "XY Chart Buffer_PINK.vi"("clear first (no:F)"=w294, "chart length (points)"=10000, "YNew"=w295, "XNew"=w297) -> ("Value Y"=w305:dbl[], "Value X"=w304:dbl[])  [unwired: 6 in]
          n108 = Bundle("Value X"=w304, "Value Y"=w305) -> (w303:cluster{"Value X":dbl[], "Value Y":dbl[]})  [unwired: 1 in]
          n109 = Build Array(w303) -> (w298:cluster{"Value X":dbl[], "Value Y":dbl[]}[])
          n110 = property class="XYGraph (strict)"(reference=w292, "Value"=w298, "XScale.NameLbl.Text"="Z Distance (um)" ("X Scale.Name Label.Text"), "YScale.NameLbl.Text"="Current 3 (nA)" ("Y Scale.Name Label.Text"), "YScale.Multiplier"=1000000000.0 ("Y Scale.Offset and Multiplier:Multiplier")) -> ()  [unwired: 1 in, 2 out]
        }
        frame True {
        }
      }
    }
    frame #18 {
      # "V vs C1"
      n111 = Not A Number/Path/Refnum?(number/path/refnum=w308) -> (NaN/Path/Refnum?=w309:bool)
      n112 = case shown="False" w309 {
        tunnel: w308 -> [w315 _]
        tunnel: w307 -> [w314 _]
        tunnel: w306 -> [w313 _]
        frame False {
          n113 = Index Array ("Oscillation Amplitude")(array=w314, index (row)=3 ("disabled index (row)"), index (col)=0) -> (element=w318:dbl)
          n114 = Index Array ("Oscillation Amplitude")(array=w314, index (row)=5 ("disabled index (row)"), index (col)=0) -> (element=w316:dbl)
          n115 = call "XY Chart Buffer_PINK.vi"("clear first (no:F)"=w313, "chart length (points)"=10000, "YNew"=w316, "XNew"=w318) -> ("Value Y"=w326:dbl[], "Value X"=w325:dbl[])  [unwired: 6 in]
          n116 = Bundle("Value X"=w325, "Value Y"=w326) -> (w324:cluster{"Value X":dbl[], "Value Y":dbl[]})  [unwired: 1 in]
          n117 = Build Array(w324) -> (w319:cluster{"Value X":dbl[], "Value Y":dbl[]}[])
          n118 = property class="XYGraph (strict)"(reference=w315, "Value"=w319, "XScale.NameLbl.Text"="Potential (V)" ("X Scale.Name Label.Text"), "YScale.NameLbl.Text"="Current 1 (nA)" ("Y Scale.Name Label.Text"), "YScale.Multiplier"=1000000000.0 ("Y Scale.Offset and Multiplier:Multiplier")) -> ()  [unwired: 1 in, 2 out]
        }
        frame True {
        }
      }
    }
    frame #19 {
      # "V vs C2"
      n119 = Not A Number/Path/Refnum?(number/path/refnum=w327) -> (NaN/Path/Refnum?=w330:bool)
      n120 = case shown="False" w330 {
        tunnel: w329 -> [w336 _]
        tunnel: w328 -> [w335 _]
        tunnel: w327 -> [w334 _]
        frame False {
          n121 = Index Array ("Oscillation Amplitude")(array=w336, index (row)=3 ("disabled index (row)"), index (col)=0) -> (element=w339:dbl)
          n122 = Index Array ("Oscillation Amplitude")(array=w336, index (row)=6 ("disabled index (row)"), index (col)=0) -> (element=w337:dbl)
          n123 = call "XY Chart Buffer_PINK.vi"("clear first (no:F)"=w335, "chart length (points)"=10000, "YNew"=w337, "XNew"=w339) -> ("Value Y"=w347:dbl[], "Value X"=w346:dbl[])  [unwired: 6 in]
          n124 = Bundle("Value X"=w346, "Value Y"=w347) -> (w345:cluster{"Value X":dbl[], "Value Y":dbl[]})  [unwired: 1 in]
          n125 = Build Array(w345) -> (w340:cluster{"Value X":dbl[], "Value Y":dbl[]}[])
          n126 = property class="XYGraph (strict)"(reference=w334, "Value"=w340, "XScale.NameLbl.Text"="Potential (V)" ("X Scale.Name Label.Text"), "YScale.NameLbl.Text"="Current 2 (nA)" ("Y Scale.Name Label.Text"), "YScale.Multiplier"=1000000000.0 ("Y Scale.Offset and Multiplier:Multiplier")) -> ()  [unwired: 1 in, 2 out]
        }
        frame True {
        }
      }
    }
    frame #20 {
      # "V vs C3"
      n127 = Not A Number/Path/Refnum?(number/path/refnum=w349) -> (NaN/Path/Refnum?=w351:bool)
      n128 = case shown="False" w351 {
        tunnel: w350 -> [w357 _]
        tunnel: w349 -> [w356 _]
        tunnel: w348 -> [w355 _]
        frame False {
          n129 = Index Array ("Oscillation Amplitude")(array=w355, index (row)=3 ("disabled index (row)"), index (col)=0) -> (element=w366:dbl)
          n130 = Index Array ("Oscillation Amplitude")(array=w355, index (row)=7 ("disabled index (row)"), index (col)=0) -> (element=w368:dbl)
          n131 = call "XY Chart Buffer_PINK.vi"("clear first (no:F)"=w357, "chart length (points)"=10000, "YNew"=w368, "XNew"=w366) -> ("Value Y"=w358:dbl[], "Value X"=w359:dbl[])  [unwired: 6 in]
          n132 = Bundle("Value X"=w359, "Value Y"=w358) -> (w360:cluster{"Value X":dbl[], "Value Y":dbl[]})  [unwired: 1 in]
          n133 = Build Array(w360) -> (w365:cluster{"Value X":dbl[], "Value Y":dbl[]}[])
          n134 = property class="XYGraph (strict)"(reference=w356, "Value"=w365, "XScale.NameLbl.Text"="Potential (V)" ("X Scale.Name Label.Text"), "YScale.NameLbl.Text"="Current 3 (nA)" ("Y Scale.Name Label.Text"), "YScale.Multiplier"=1000000000.0 ("Y Scale.Offset and Multiplier:Multiplier")) -> ()  [unwired: 1 in, 2 out]
        }
        frame True {
        }
      }
    }
    frame #21 {
      # "X/Y/Z"
      n135 = Not A Number/Path/Refnum?(number/path/refnum=w375) -> (NaN/Path/Refnum?=w373:bool)
      n136 = Not A Number/Path/Refnum?(number/path/refnum=w376) -> (NaN/Path/Refnum?=w374:bool)
      n137 = Not(x=w373) -> (.not. x?=w369:bool)
      n138 = Not(x=w374) -> (.not. x?=w370:bool)
      n139 = Or(x=w370, y=w369) -> (x .or. y?=w372:bool)
      n140 = case shown="True" w372 {
        tunnel: w371 -> [_ w381]
        frame False {
        }
        frame True {
          n141 = Index Array "Feedback type"(array=w381, index (row)=8, index (col)=0 ("disabled index (col)")) -> (element=w379:dbl)
          n142 = Equal?(x=w379, y=4.0) -> (x = y?=w380:bool)
          n143 = case shown="True" w380 {
            tunnel: w381 -> [_ w389]
            tunnel: [TRUE w388] -> w377
            frame False {
            }
            frame True {
              n144 = global read "Settings.vi" "Waypoints per hop"() -> (w387:dbl)
              n145 = Equal?(x=w387, y=4.0) -> (x = y?=w385:bool)
              n146 = case shown="False" w385 {
                tunnel: w389 -> [w404 w480]
                tunnel: [w403 w479] -> w388
                frame False {
                  w400 = 2.0 ("disabled index (col)")
                  n147 = local read "Display Cluster"() -> (w402:T1)
                  n148 = local read "Topology"() -> (w422:bool)
                  n149 = Unbundle By Name(w402) -> ("um Per Line"=w392:dbl, "um Per Pixel"=w394:dbl, "NumberOfLines"=w407:u16, "X/Y/Z F"=w409:refnum<vi>, "X/Y/Z R"=w408:refnum<vi>, "X Center"=w398:dbl, "X Width"=w390:dbl, "Y Width"=w396:dbl, "Y Center"=w395:dbl, "Number of Pixels"=w391:dbl)
                  n150 = Index Array "LineNumber"(array=w404, index (row)=9 ("disabled index (row)"), index (col)=0 ("disabled index (col)")) -> (element=w425:dbl)
                  n151 = case shown="True" w422 {
                    tunnel: w407 -> [_ w440]
                    tunnel: [FALSE FALSE] -> w403
                    tunnel: [w432 w435] -> w406
                    tunnel: [w431 w435] -> w405
                    tunnel: w404 -> [_ w439]
                    tunnel: w391 -> [_ w434]
                    frame False {
                      n152 = local read "Forward Topo"() -> (w432:dbl[][])
                      n153 = local read "Reverse Topo"() -> (w431:dbl[][])
                    }
                    frame True {
                      n154 = Index Array "Z"(array=w439, index (row)=2 ("disabled index (row)"), index (col)=0 ("disabled index (col)")) -> (element=w436:dbl)
                      n155 = Initialize Array(w436, w434, w440) -> (w435:dbl[][])
                    }
                  }
                  n156 = Subtract(x=w425, y=4.0) -> (x-y=w423:dbl)
                  n157 = Quotient & Remainder(x=w423, y=6.0) -> (x-y*floor(x/y)=w427:dbl, floor(x/y)=w426:dbl)
                  n158 = Divide(x=w390, y=w400) -> (x/y=w401:dbl)
                  n159 = Divide(x=w396, y=w400) -> (x/y=w399:dbl)
                  n160 = Subtract(x=w398, y=w401) -> (x-y=w397:dbl)
                  n161 = Subtract(x=w395, y=w399) -> (x-y=w393:dbl)
                  n162 = local write "Reverse Topo"(w405) -> ()
                  n163 = Divide(x=w390, y=2.0) -> (x/y=w420:dbl)
                  n164 = Index Array "X"(array=w404, index (row)=0 ("disabled index (row)"), index (col)=0 ("disabled index (col)")) -> (element=w417:dbl)
                  n165 = Subtract(x=w398, y=w420) -> (x-y=w416:dbl)
                  n166 = Subtract(x=w417, y=w416) -> (x-y=w415:dbl)
                  n167 = Divide(x=w415, y=w394) -> (x/y=w414:dbl)
                  n168 = local write "Forward Topo"(w406) -> ()
                  n169 = Round Toward -Infinity(1:w414) -> (0:w413:dbl)
                  n170 = Index Array "Z"(array=w404, index (row)=2 ("disabled index (row)"), index (col)=0 ("disabled index (col)")) -> (element=w410:dbl)
                  n171 = case shown="0, Default" w427 {
                    tunnel: w426 -> [w449 w459]
                    tunnel: w413 -> [w450 w457]
                    tunnel: w406 -> [w451 _]
                    tunnel: w405 -> [_ w461]
                    tunnel: w410 -> [w448 w460]
                    tunnel: w409 -> [w446 _]
                    tunnel: w408 -> [_ w456]
                    tunnel: w397 -> [w445 w455]
                    tunnel: w394 -> [w444 w453]
                    tunnel: w393 -> [w443 w454]
                    tunnel: w392 -> [w442 w452]
                    frame 0, Default {
                      n172 = Replace Array Subset(array=w451, new element=w448, index (row)=w450, index (col)=w449) -> (w447:dbl[][])
                      "Forward Topo" <- w447
                      n173 = property class="IntGraph (strict)"(reference=w446, "Value"=w447, "XScale.Offset"=w445, "XScale.Multiplier"=w444, "YScale.Offset"=w443, "YScale.Multiplier"=w442) -> ()  [unwired: 1 in, 2 out]
                    }
                    frame 2 {
                      n174 = Replace Array Subset(array=w461, new element=w460, index (row)=w457, index (col)=w459) -> (w458:dbl[][])
                      "Reverse Topo" <- w458
                      n175 = property class="IntGraph (strict)"(reference=w456, "Value"=w458, "XScale.Offset"=w455, "XScale.Multiplier"=w453, "YScale.Offset"=w454, "YScale.Multiplier"=w452) -> ()  [unwired: 1 in, 2 out]
                    }
                  }
                }
                frame True {
                  w476 = 2.0 ("disabled index (col)")
                  n176 = local read "Display Cluster"() -> (w478:T1)
                  n177 = local read "Topology"() -> (w496:bool)
                  n178 = Unbundle By Name(w478) -> ("um Per Line"=w469:dbl, "um Per Pixel"=w471:dbl, "NumberOfLines"=w482:u16, "X/Y/Z F"=w483:refnum<vi>, "X Center"=w474:dbl, "X Width"=w467:dbl, "Y Width"=w462:dbl, "Y Center"=w472:dbl, "Number of Pixels"=w468:dbl)
                  n179 = Index Array "LineNumber"(array=w480, index (row)=9 ("disabled index (row)"), index (col)=0 ("disabled index (col)")) -> (element=w498:dbl)
                  n180 = case shown="True" w496 {
                    tunnel: w482 -> [_ w509]
                    tunnel: [FALSE FALSE] -> w479
                    tunnel: [w501 w504] -> w481
                    tunnel: w480 -> [_ w508]
                    tunnel: w468 -> [_ w503]
                    frame False {
                      n181 = local read "Raster Topo"() -> (w501:dbl[][])
                    }
                    frame True {
                      n182 = Index Array "Z"(array=w508, index (row)=2 ("disabled index (row)"), index (col)=0 ("disabled index (col)")) -> (element=w505:dbl)
                      n183 = Initialize Array(w505, w503, w509) -> (w504:dbl[][])
                    }
                  }
                  n184 = Subtract(x=w498, y=2.0) -> (x-y=w464:dbl)
                  n185 = Divide(x=w464, y=4.0) -> (x/y=w465:dbl)
                  n186 = Divide(x=w467, y=w476) -> (x/y=w477:dbl)
                  n187 = Divide(x=w462, y=w476) -> (x/y=w475:dbl)
                  n188 = Subtract(x=w474, y=w477) -> (x-y=w473:dbl)
                  n189 = Subtract(x=w472, y=w475) -> (x-y=w470:dbl)
                  n190 = Divide(x=w467, y=2.0) -> (x/y=w494:dbl)
                  n191 = Index Array "X"(array=w480, index (row)=0 ("disabled index (row)"), index (col)=0 ("disabled index (col)")) -> (element=w491:dbl)
                  n192 = Subtract(x=w474, y=w494) -> (x-y=w490:dbl)
                  n193 = Subtract(x=w491, y=w490) -> (x-y=w489:dbl)
                  n194 = Divide(x=w489, y=w471) -> (x/y=w488:dbl)
                  n195 = local write "Raster Topo"(w481) -> ()
                  n196 = Round Toward -Infinity(1:w488) -> (0:w487:dbl)
                  n197 = Index Array "Z"(array=w480, index (row)=2 ("disabled index (row)"), index (col)=0 ("disabled index (col)")) -> (element=w484:dbl)
                  n198 = Replace Array Subset(array=w481, new element=w484, index (row)=w487, index (col)=w465) -> (w466:dbl[][])
                  "Raster Topo" <- w466
                  n199 = property class="IntGraph (strict)"(reference=w483, "Value"=w466, "XScale.Offset"=w473, "XScale.Multiplier"=w471, "YScale.Offset"=w470, "YScale.Multiplier"=w469) -> ()  [unwired: 1 in, 2 out]
                }
              }
            }
          }
          "Topology" <- w377
        }
      }
    }
    frame #22 {
      # "X/Y/C1"
      n200 = Not A Number/Path/Refnum?(number/path/refnum=w513) -> (NaN/Path/Refnum?=w517:bool)
      n201 = Not A Number/Path/Refnum?(number/path/refnum=w514) -> (NaN/Path/Refnum?=w518:bool)
      n202 = Not(x=w518) -> (.not. x?=w512:bool)
      n203 = Not(x=w517) -> (.not. x?=w511:bool)
      n204 = Or(x=w512, y=w511) -> (x .or. y?=w516:bool)
      n205 = case shown="True" w516 {
        tunnel: w515 -> [_ w523]
        frame False {
        }
        frame True {
          n206 = Index Array "Feedback type"(array=w523, index (row)=8, index (col)=0 ("disabled index (col)")) -> (element=w521:dbl)
          n207 = Equal?(x=w521, y=4.0) -> (x = y?=w522:bool)
          n208 = case shown="True" w522 {
            tunnel: w523 -> [_ w531]
            tunnel: [TRUE w530] -> w519
            frame False {
            }
            frame True {
              n209 = global read "Settings.vi" "Waypoints per hop"() -> (w529:dbl)
              n210 = Equal?(x=w529, y=4.0) -> (x = y?=w527:bool)
              n211 = case shown="True" w527 {
                tunnel: w531 -> [w547 w623]
                tunnel: [w546 w622] -> w530
                frame False {
                  w543 = 2.0 ("disabled index (col)")
                  n212 = local read "Display Cluster"() -> (w545:T1)
                  n213 = local read "Current 1"() -> (w532:bool)
                  n214 = Unbundle By Name(w545) -> ("um Per Line"=w535:dbl, "um Per Pixel"=w537:dbl, "NumberOfLines"=w550:u16, "X/Y/C1 F"=w552:refnum<vi>, "X/Y/C1 R"=w551:refnum<vi>, "X Center"=w541:dbl, "X Width"=w533:dbl, "Y Width"=w539:dbl, "Y Center"=w538:dbl, "Number of Pixels"=w534:dbl)
                  n215 = Index Array "LineNumber"(array=w547, index (row)=9 ("disabled index (row)"), index (col)=0 ("disabled index (col)")) -> (element=w567:dbl)
                  n216 = case shown="True" w532 {
                    tunnel: w550 -> [_ w582]
                    tunnel: [FALSE FALSE] -> w546
                    tunnel: [w574 w577] -> w549
                    tunnel: [w573 w577] -> w548
                    tunnel: w547 -> [_ w581]
                    tunnel: w534 -> [_ w576]
                    frame False {
                      n217 = local read "Forward Current1"() -> (w574:dbl[][])
                      n218 = local read "Reverse Current1"() -> (w573:dbl[][])
                    }
                    frame True {
                      n219 = Index Array "C1"(array=w581, index (row)=5 ("disabled index (row)"), index (col)=0 ("disabled index (col)")) -> (element=w578:dbl)
                      n220 = Initialize Array(w578, w576, w582) -> (w577:dbl[][])
                    }
                  }
                  n221 = Subtract(x=w567, y=4.0) -> (x-y=w565:dbl)
                  n222 = Quotient & Remainder(x=w565, y=6.0) -> (x-y*floor(x/y)=w569:dbl, floor(x/y)=w568:dbl)
                  n223 = Divide(x=w533, y=w543) -> (x/y=w544:dbl)
                  n224 = Divide(x=w539, y=w543) -> (x/y=w542:dbl)
                  n225 = Subtract(x=w541, y=w544) -> (x-y=w540:dbl)
                  n226 = Subtract(x=w538, y=w542) -> (x-y=w536:dbl)
                  n227 = local write "Reverse Current1"(w548) -> ()
                  n228 = Divide(x=w533, y=2.0) -> (x/y=w563:dbl)
                  n229 = Index Array "X"(array=w547, index (row)=0 ("disabled index (row)"), index (col)=0 ("disabled index (col)")) -> (element=w560:dbl)
                  n230 = Subtract(x=w541, y=w563) -> (x-y=w559:dbl)
                  n231 = Subtract(x=w560, y=w559) -> (x-y=w558:dbl)
                  n232 = Divide(x=w558, y=w537) -> (x/y=w557:dbl)
                  n233 = local write "Forward Current1"(w549) -> ()
                  n234 = Round Toward -Infinity(1:w557) -> (0:w556:dbl)
                  n235 = Index Array "C1"(array=w547, index (row)=5 ("disabled index (row)"), index (col)=0 ("disabled index (col)")) -> (element=w553:dbl)
                  n236 = case shown="2" w569 {
                    tunnel: w568 -> [w591 w601]
                    tunnel: w556 -> [w592 w600]
                    tunnel: w549 -> [w593 _]
                    tunnel: w548 -> [_ w603]
                    tunnel: w553 -> [w590 w602]
                    tunnel: w552 -> [w589 _]
                    tunnel: w551 -> [_ w599]
                    tunnel: w540 -> [w588 w598]
                    tunnel: w537 -> [w587 w596]
                    tunnel: w536 -> [w586 w597]
                    tunnel: w535 -> [w585 w595]
                    frame 0, Default {
                      n237 = Replace Array Subset(array=w593, new element=w590, index (row)=w592, index (col)=w591) -> (w584:dbl[][])
                      "Forward Current1" <- w584
                      n238 = property class="IntGraph (strict)"(reference=w589, "Value"=w584, "XScale.Offset"=w588, "XScale.Multiplier"=w587, "YScale.Offset"=w586, "YScale.Multiplier"=w585) -> ()  [unwired: 1 in, 2 out]
                    }
                    frame 2 {
                      n239 = Replace Array Subset(array=w603, new element=w602, index (row)=w600, index (col)=w601) -> (w594:dbl[][])
                      "Reverse Current1" <- w594
                      n240 = property class="IntGraph (strict)"(reference=w599, "Value"=w594, "XScale.Offset"=w598, "XScale.Multiplier"=w596, "YScale.Offset"=w597, "YScale.Multiplier"=w595) -> ()  [unwired: 1 in, 2 out]
                    }
                  }
                }
                frame True {
                  w619 = 2.0 ("disabled index (col)")
                  n241 = local read "Display Cluster"() -> (w621:T1)
                  n242 = local read "Current 1"() -> (w604:bool)
                  n243 = Unbundle By Name(w621) -> ("um Per Line"=w611:dbl, "um Per Pixel"=w613:dbl, "NumberOfLines"=w625:u16, "X/Y/C1 F"=w626:refnum<vi>, "X Center"=w617:dbl, "X Width"=w609:dbl, "Y Width"=w615:dbl, "Y Center"=w614:dbl, "Number of Pixels"=w610:dbl)
                  n244 = Index Array "LineNumber"(array=w623, index (row)=9 ("disabled index (row)"), index (col)=0 ("disabled index (col)")) -> (element=w640:dbl)
                  n245 = case shown="True" w604 {
                    tunnel: w625 -> [_ w651]
                    tunnel: [FALSE FALSE] -> w622
                    tunnel: [w643 w646] -> w624
                    tunnel: w623 -> [_ w650]
                    tunnel: w610 -> [_ w645]
                    frame False {
                      n246 = local read "Raster Current1"() -> (w643:dbl[][])
                    }
                    frame True {
                      n247 = Index Array "C1"(array=w650, index (row)=5 ("disabled index (row)"), index (col)=0 ("disabled index (col)")) -> (element=w647:dbl)
                      n248 = Initialize Array(w647, w645, w651) -> (w646:dbl[][])
                    }
                  }
                  n249 = Subtract(x=w640, y=2.0) -> (x-y=w606:dbl)
                  n250 = Divide(x=w606, y=4.0) -> (x/y=w607:dbl)
                  n251 = Divide(x=w609, y=w619) -> (x/y=w620:dbl)
                  n252 = Divide(x=w615, y=w619) -> (x/y=w618:dbl)
                  n253 = Subtract(x=w617, y=w620) -> (x-y=w616:dbl)
                  n254 = Subtract(x=w614, y=w618) -> (x-y=w612:dbl)
                  n255 = Divide(x=w609, y=2.0) -> (x/y=w637:dbl)
                  n256 = Index Array "X"(array=w623, index (row)=0 ("disabled index (row)"), index (col)=0 ("disabled index (col)")) -> (element=w634:dbl)
                  n257 = Subtract(x=w617, y=w637) -> (x-y=w633:dbl)
                  n258 = Subtract(x=w634, y=w633) -> (x-y=w632:dbl)
                  n259 = Divide(x=w632, y=w613) -> (x/y=w631:dbl)
                  n260 = local write "Raster Current1"(w624) -> ()
                  n261 = Round Toward -Infinity(1:w631) -> (0:w630:dbl)
                  n262 = Index Array "C1"(array=w623, index (row)=5 ("disabled index (row)"), index (col)=0 ("disabled index (col)")) -> (element=w627:dbl)
                  n263 = Replace Array Subset(array=w624, new element=w627, index (row)=w630, index (col)=w607) -> (w608:dbl[][])
                  "Raster Current1" <- w608
                  n264 = property class="IntGraph (strict)"(reference=w626, "Value"=w608, "XScale.Offset"=w616, "XScale.Multiplier"=w613, "YScale.Offset"=w612, "YScale.Multiplier"=w611) -> ()  [unwired: 1 in, 2 out]
                }
              }
            }
          }
          "Current 1" <- w519
        }
      }
    }
    frame #23 {
      # "X/Y/C2"
      n265 = Not A Number/Path/Refnum?(number/path/refnum=w655) -> (NaN/Path/Refnum?=w659:bool)
      n266 = Not A Number/Path/Refnum?(number/path/refnum=w656) -> (NaN/Path/Refnum?=w660:bool)
      n267 = Not(x=w659) -> (.not. x?=w653:bool)
      n268 = Not(x=w660) -> (.not. x?=w654:bool)
      n269 = Or(x=w654, y=w653) -> (x .or. y?=w658:bool)
      n270 = case shown="True" w658 {
        tunnel: w657 -> [_ w665]
        frame False {
        }
        frame True {
          n271 = Index Array "Feedback type"(array=w665, index (row)=8, index (col)=0 ("disabled index (col)")) -> (element=w663:dbl)
          n272 = Equal?(x=w663, y=4.0) -> (x = y?=w664:bool)
          n273 = case shown="True" w664 {
            tunnel: w665 -> [_ w673]
            tunnel: [TRUE w672] -> w661
            frame False {
            }
            frame True {
              n274 = global read "Settings.vi" "Waypoints per hop"() -> (w671:dbl)
              n275 = Equal?(x=w671, y=4.0) -> (x = y?=w669:bool)
              n276 = case shown="False" w669 {
                tunnel: w673 -> [w689 w765]
                tunnel: [w688 w764] -> w672
                frame False {
                  w685 = 2.0 ("disabled index (col)")
                  n277 = local read "Display Cluster"() -> (w687:T1)
                  n278 = local read "Current 2"() -> (w674:bool)
                  n279 = Unbundle By Name(w687) -> ("um Per Line"=w677:dbl, "um Per Pixel"=w679:dbl, "NumberOfLines"=w692:u16, "X/Y/C2 F"=w694:refnum<vi>, "X/Y/C2 R"=w693:refnum<vi>, "X Center"=w683:dbl, "X Width"=w675:dbl, "Y Width"=w681:dbl, "Y Center"=w680:dbl, "Number of Pixels"=w676:dbl)
                  n280 = Index Array "LineNumber"(array=w689, index (row)=9 ("disabled index (row)"), index (col)=0 ("disabled index (col)")) -> (element=w709:dbl)
                  n281 = case shown="True" w674 {
                    tunnel: w692 -> [_ w724]
                    tunnel: [FALSE FALSE] -> w688
                    tunnel: [w716 w719] -> w691
                    tunnel: [w715 w719] -> w690
                    tunnel: w689 -> [_ w723]
                    tunnel: w676 -> [_ w718]
                    frame False {
                      n282 = local read "Forward Current2"() -> (w716:dbl[][])
                      n283 = local read "Reverse Current2"() -> (w715:dbl[][])
                    }
                    frame True {
                      n284 = Index Array "C2"(array=w723, index (row)=6 ("disabled index (row)"), index (col)=0 ("disabled index (col)")) -> (element=w720:dbl)
                      n285 = Initialize Array(w720, w718, w724) -> (w719:dbl[][])
                    }
                  }
                  n286 = Subtract(x=w709, y=4.0) -> (x-y=w707:dbl)
                  n287 = Quotient & Remainder(x=w707, y=6.0) -> (x-y*floor(x/y)=w711:dbl, floor(x/y)=w710:dbl)
                  n288 = Divide(x=w675, y=w685) -> (x/y=w686:dbl)
                  n289 = Divide(x=w681, y=w685) -> (x/y=w684:dbl)
                  n290 = Subtract(x=w683, y=w686) -> (x-y=w682:dbl)
                  n291 = Subtract(x=w680, y=w684) -> (x-y=w678:dbl)
                  n292 = local write "Reverse Current2"(w690) -> ()
                  n293 = Divide(x=w675, y=2.0) -> (x/y=w705:dbl)
                  n294 = Index Array "X"(array=w689, index (row)=0 ("disabled index (row)"), index (col)=0 ("disabled index (col)")) -> (element=w702:dbl)
                  n295 = Subtract(x=w683, y=w705) -> (x-y=w701:dbl)
                  n296 = Subtract(x=w702, y=w701) -> (x-y=w700:dbl)
                  n297 = Divide(x=w700, y=w679) -> (x/y=w699:dbl)
                  n298 = local write "Forward Current2"(w691) -> ()
                  n299 = Round Toward -Infinity(1:w699) -> (0:w698:dbl)
                  n300 = Index Array "C2"(array=w689, index (row)=6 ("disabled index (row)"), index (col)=0 ("disabled index (col)")) -> (element=w695:dbl)
                  n301 = case shown="0, Default" w711 {
                    tunnel: w710 -> [w733 w743]
                    tunnel: w698 -> [w734 w742]
                    tunnel: w691 -> [w735 _]
                    tunnel: w690 -> [_ w745]
                    tunnel: w695 -> [w732 w744]
                    tunnel: w694 -> [w731 _]
                    tunnel: w693 -> [_ w741]
                    tunnel: w682 -> [w730 w740]
                    tunnel: w679 -> [w729 w738]
                    tunnel: w678 -> [w728 w739]
                    tunnel: w677 -> [w727 w737]
                    frame 0, Default {
                      n302 = Replace Array Subset(array=w735, new element=w732, index (row)=w734, index (col)=w733) -> (w726:dbl[][])
                      "Forward Current2" <- w726
                      n303 = property class="IntGraph (strict)"(reference=w731, "Value"=w726, "XScale.Offset"=w730, "XScale.Multiplier"=w729, "YScale.Offset"=w728, "YScale.Multiplier"=w727) -> ()  [unwired: 1 in, 2 out]
                    }
                    frame 2 {
                      n304 = Replace Array Subset(array=w745, new element=w744, index (row)=w742, index (col)=w743) -> (w736:dbl[][])
                      "Reverse Current2" <- w736
                      n305 = property class="IntGraph (strict)"(reference=w741, "Value"=w736, "XScale.Offset"=w740, "XScale.Multiplier"=w738, "YScale.Offset"=w739, "YScale.Multiplier"=w737) -> ()  [unwired: 1 in, 2 out]
                    }
                  }
                }
                frame True {
                  w761 = 2.0 ("disabled index (col)")
                  n306 = local read "Display Cluster"() -> (w763:T1)
                  n307 = local read "Current 2"() -> (w746:bool)
                  n308 = Unbundle By Name(w763) -> ("um Per Line"=w753:dbl, "um Per Pixel"=w755:dbl, "NumberOfLines"=w767:u16, "X/Y/C2 F"=w768:refnum<vi>, "X Center"=w759:dbl, "X Width"=w751:dbl, "Y Width"=w757:dbl, "Y Center"=w756:dbl, "Number of Pixels"=w752:dbl)
                  n309 = Index Array "LineNumber"(array=w765, index (row)=9 ("disabled index (row)"), index (col)=0 ("disabled index (col)")) -> (element=w782:dbl)
                  n310 = case shown="True" w746 {
                    tunnel: w767 -> [_ w793]
                    tunnel: [FALSE FALSE] -> w764
                    tunnel: [w785 w788] -> w766
                    tunnel: w765 -> [_ w792]
                    tunnel: w752 -> [_ w787]
                    frame False {
                      n311 = local read "Raster Current 2"() -> (w785:dbl[][])
                    }
                    frame True {
                      n312 = Index Array "C2"(array=w792, index (row)=6 ("disabled index (row)"), index (col)=0 ("disabled index (col)")) -> (element=w789:dbl)
                      n313 = Initialize Array(w789, w787, w793) -> (w788:dbl[][])
                    }
                  }
                  n314 = Subtract(x=w782, y=2.0) -> (x-y=w748:dbl)
                  n315 = Divide(x=w748, y=4.0) -> (x/y=w749:dbl)
                  n316 = Divide(x=w751, y=w761) -> (x/y=w762:dbl)
                  n317 = Divide(x=w757, y=w761) -> (x/y=w760:dbl)
                  n318 = Subtract(x=w759, y=w762) -> (x-y=w758:dbl)
                  n319 = Subtract(x=w756, y=w760) -> (x-y=w754:dbl)
                  n320 = Divide(x=w751, y=2.0) -> (x/y=w779:dbl)
                  n321 = Index Array "X"(array=w765, index (row)=0 ("disabled index (row)"), index (col)=0 ("disabled index (col)")) -> (element=w776:dbl)
                  n322 = Subtract(x=w759, y=w779) -> (x-y=w775:dbl)
                  n323 = Subtract(x=w776, y=w775) -> (x-y=w774:dbl)
                  n324 = Divide(x=w774, y=w755) -> (x/y=w773:dbl)
                  n325 = local write "Raster Current 2"(w766) -> ()
                  n326 = Round Toward -Infinity(1:w773) -> (0:w772:dbl)
                  n327 = Index Array "C2"(array=w765, index (row)=6 ("disabled index (row)"), index (col)=0 ("disabled index (col)")) -> (element=w769:dbl)
                  n328 = Replace Array Subset(array=w766, new element=w769, index (row)=w772, index (col)=w749) -> (w750:dbl[][])
                  "Raster Current 2" <- w750
                  n329 = property class="IntGraph (strict)"(reference=w768, "Value"=w750, "XScale.Offset"=w758, "XScale.Multiplier"=w755, "YScale.Offset"=w754, "YScale.Multiplier"=w753) -> ()  [unwired: 1 in, 2 out]
                }
              }
            }
          }
          "Current 2" <- w661
        }
      }
    }
    frame #24 {
      # "X/Y/C3"
      n330 = Not A Number/Path/Refnum?(number/path/refnum=w797) -> (NaN/Path/Refnum?=w801:bool)
      n331 = Not A Number/Path/Refnum?(number/path/refnum=w798) -> (NaN/Path/Refnum?=w802:bool)
      n332 = Not(x=w802) -> (.not. x?=w796:bool)
      n333 = Not(x=w801) -> (.not. x?=w795:bool)
      n334 = Or(x=w796, y=w795) -> (x .or. y?=w800:bool)
      n335 = case shown="True" w800 {
        tunnel: w799 -> [_ w807]
        frame False {
        }
        frame True {
          n336 = Index Array "Feedback type"(array=w807, index (row)=8, index (col)=0 ("disabled index (col)")) -> (element=w805:dbl)
          n337 = Equal?(x=w805, y=4.0) -> (x = y?=w806:bool)
          n338 = case shown="True" w806 {
            tunnel: w807 -> [_ w815]
            tunnel: [TRUE w814] -> w803
            frame False {
            }
            frame True {
              n339 = global read "Settings.vi" "Waypoints per hop"() -> (w813:dbl)
              n340 = Equal?(x=w813, y=4.0) -> (x = y?=w811:bool)
              n341 = case shown="True" w811 {
                tunnel: w815 -> [w831 w907]
                tunnel: [w830 w906] -> w814
                frame False {
                  w827 = 2.0 ("disabled index (col)")
                  n342 = local read "Display Cluster"() -> (w829:T1)
                  n343 = local read "Current 3"() -> (w816:bool)
                  n344 = Unbundle By Name(w829) -> ("um Per Line"=w819:dbl, "um Per Pixel"=w821:dbl, "NumberOfLines"=w834:u16, "X/Y/C3 F"=w836:refnum<vi>, "X/Y/C3 R"=w835:refnum<vi>, "X Center"=w825:dbl, "X Width"=w817:dbl, "Y Width"=w823:dbl, "Y Center"=w822:dbl, "Number of Pixels"=w818:dbl)
                  n345 = Index Array "LineNumber"(array=w831, index (row)=9 ("disabled index (row)"), index (col)=0 ("disabled index (col)")) -> (element=w851:dbl)
                  n346 = case shown="True" w816 {
                    tunnel: w834 -> [_ w866]
                    tunnel: [FALSE FALSE] -> w830
                    tunnel: [w858 w861] -> w833
                    tunnel: [w857 w861] -> w832
                    tunnel: w831 -> [_ w865]
                    tunnel: w818 -> [_ w860]
                    frame False {
                      n347 = local read "Forward Current3"() -> (w858:dbl[][])
                      n348 = local read "Reverse Current3"() -> (w857:dbl[][])
                    }
                    frame True {
                      n349 = Index Array "C3"(array=w865, index (row)=7 ("disabled index (row)"), index (col)=0 ("disabled index (col)")) -> (element=w862:dbl)
                      n350 = Initialize Array(w862, w860, w866) -> (w861:dbl[][])
                    }
                  }
                  n351 = Subtract(x=w851, y=4.0) -> (x-y=w849:dbl)
                  n352 = Quotient & Remainder(x=w849, y=6.0) -> (x-y*floor(x/y)=w853:dbl, floor(x/y)=w852:dbl)
                  n353 = Divide(x=w817, y=w827) -> (x/y=w828:dbl)
                  n354 = Divide(x=w823, y=w827) -> (x/y=w826:dbl)
                  n355 = Subtract(x=w825, y=w828) -> (x-y=w824:dbl)
                  n356 = Subtract(x=w822, y=w826) -> (x-y=w820:dbl)
                  n357 = local write "Reverse Current3"(w832) -> ()
                  n358 = Divide(x=w817, y=2.0) -> (x/y=w847:dbl)
                  n359 = Index Array "X"(array=w831, index (row)=0 ("disabled index (row)"), index (col)=0 ("disabled index (col)")) -> (element=w844:dbl)
                  n360 = Subtract(x=w825, y=w847) -> (x-y=w843:dbl)
                  n361 = Subtract(x=w844, y=w843) -> (x-y=w842:dbl)
                  n362 = Divide(x=w842, y=w821) -> (x/y=w841:dbl)
                  n363 = local write "Forward Current3"(w833) -> ()
                  n364 = Round Toward -Infinity(1:w841) -> (0:w840:dbl)
                  n365 = Index Array "C3"(array=w831, index (row)=7 ("disabled index (row)"), index (col)=0 ("disabled index (col)")) -> (element=w837:dbl)
                  n366 = case shown="0, Default" w853 {
                    tunnel: w852 -> [w875 w885]
                    tunnel: w840 -> [w876 w884]
                    tunnel: w833 -> [w877 _]
                    tunnel: w832 -> [_ w887]
                    tunnel: w837 -> [w874 w886]
                    tunnel: w836 -> [w873 _]
                    tunnel: w835 -> [_ w883]
                    tunnel: w824 -> [w872 w882]
                    tunnel: w821 -> [w871 w880]
                    tunnel: w820 -> [w870 w881]
                    tunnel: w819 -> [w869 w879]
                    frame 0, Default {
                      n367 = Replace Array Subset(array=w877, new element=w874, index (row)=w876, index (col)=w875) -> (w868:dbl[][])
                      "Forward Current3" <- w868
                      n368 = property class="IntGraph (strict)"(reference=w873, "Value"=w868, "XScale.Offset"=w872, "XScale.Multiplier"=w871, "YScale.Offset"=w870, "YScale.Multiplier"=w869) -> ()  [unwired: 1 in, 2 out]
                    }
                    frame 2 {
                      n369 = Replace Array Subset(array=w887, new element=w886, index (row)=w884, index (col)=w885) -> (w878:dbl[][])
                      "Reverse Current3" <- w878
                      n370 = property class="IntGraph (strict)"(reference=w883, "Value"=w878, "XScale.Offset"=w882, "XScale.Multiplier"=w880, "YScale.Offset"=w881, "YScale.Multiplier"=w879) -> ()  [unwired: 1 in, 2 out]
                    }
                  }
                }
                frame True {
                  w903 = 2.0 ("disabled index (col)")
                  n371 = local read "Display Cluster"() -> (w905:T1)
                  n372 = local read "Current 3"() -> (w888:bool)
                  n373 = Unbundle By Name(w905) -> ("um Per Line"=w895:dbl, "um Per Pixel"=w897:dbl, "NumberOfLines"=w909:u16, "X/Y/C3 F"=w910:refnum<vi>, "X Center"=w901:dbl, "X Width"=w893:dbl, "Y Width"=w899:dbl, "Y Center"=w898:dbl, "Number of Pixels"=w894:dbl)
                  n374 = Index Array "LineNumber"(array=w907, index (row)=9 ("disabled index (row)"), index (col)=0 ("disabled index (col)")) -> (element=w924:dbl)
                  n375 = case shown="True" w888 {
                    tunnel: w909 -> [_ w935]
                    tunnel: [FALSE FALSE] -> w906
                    tunnel: [w927 w930] -> w908
                    tunnel: w907 -> [_ w934]
                    tunnel: w894 -> [_ w929]
                    frame False {
                      n376 = local read "Raster Current 3"() -> (w927:dbl[][])
                    }
                    frame True {
                      n377 = Index Array "C3"(array=w934, index (row)=7 ("disabled index (row)"), index (col)=0 ("disabled index (col)")) -> (element=w931:dbl)
                      n378 = Initialize Array(w931, w929, w935) -> (w930:dbl[][])
                    }
                  }
                  n379 = Subtract(x=w924, y=2.0) -> (x-y=w890:dbl)
                  n380 = Divide(x=w890, y=4.0) -> (x/y=w891:dbl)
                  n381 = Divide(x=w893, y=w903) -> (x/y=w904:dbl)
                  n382 = Divide(x=w899, y=w903) -> (x/y=w902:dbl)
                  n383 = Subtract(x=w901, y=w904) -> (x-y=w900:dbl)
                  n384 = Subtract(x=w898, y=w902) -> (x-y=w896:dbl)
                  n385 = Divide(x=w893, y=2.0) -> (x/y=w921:dbl)
                  n386 = Index Array "X"(array=w907, index (row)=0 ("disabled index (row)"), index (col)=0 ("disabled index (col)")) -> (element=w918:dbl)
                  n387 = Subtract(x=w901, y=w921) -> (x-y=w917:dbl)
                  n388 = Subtract(x=w918, y=w917) -> (x-y=w916:dbl)
                  n389 = Divide(x=w916, y=w897) -> (x/y=w915:dbl)
                  n390 = local write "Raster Current 3"(w908) -> ()
                  n391 = Round Toward -Infinity(1:w915) -> (0:w914:dbl)
                  n392 = Index Array "C3"(array=w907, index (row)=7 ("disabled index (row)"), index (col)=0 ("disabled index (col)")) -> (element=w911:dbl)
                  n393 = Replace Array Subset(array=w908, new element=w911, index (row)=w914, index (col)=w891) -> (w892:dbl[][])
                  "Raster Current 3" <- w892
                  n394 = property class="IntGraph (strict)"(reference=w910, "Value"=w892, "XScale.Offset"=w900, "XScale.Multiplier"=w897, "YScale.Offset"=w896, "YScale.Multiplier"=w895) -> ()  [unwired: 1 in, 2 out]
                }
              }
            }
          }
          "Current 3" <- w803
        }
      }
    }
    frame #25 {
      # "Hop\nX/Y/Z"
      n395 = Not A Number/Path/Refnum?(number/path/refnum=w938) -> (NaN/Path/Refnum?=w937:bool)
      n396 = case shown="False" w937 {
        tunnel: w939 -> [w975 _]
        frame False {
          w943 = 2.0 ("disabled index (col)")
          # "Y only goes up\n\nX goes back and forth"
          # "If new then set the array in the shape of the graph"
          # "New scan?"
          n397 = local read "Display Cluster"() -> (w955:T1)
          n398 = Unbundle By Name(w955) -> ("Hop X/Y/Z"=w967:refnum<vi>, "X Width"=w948:dbl, "Y Width"=w944:dbl, "Hopping Distance"=w949:dbl, "X Center"=w947:dbl, "Y Center"=w940:dbl)
          n399 = Index Array "LineNumber"(array=w975, index (row)=9 ("disabled index (row)"), index (col)=0 ("disabled index (col)")) -> (element=w961:dbl)
          n400 = Equal?(x=w961, y=2.0) -> (x = y?=w959:bool)
          n401 = Select(t=TRUE, s=w959, f=FALSE) -> (s? t:f=w956:bool)
          n402 = Divide(x=w944, y=w949) -> (x/y=w963:dbl)
          n403 = Round Toward -Infinity(1:w963) -> (0:w964:dbl)
          n404 = Divide(x=w948, y=w949) -> (x/y=w969:dbl)
          n405 = local write "Hop Top"(w956) -> ()
          n406 = Increment(x=w964) -> (x+1=w962:dbl)
          n407 = Divide(x=w948, y=w943) -> (x/y=w946:dbl)
          n408 = Round Toward -Infinity(1:w969) -> (0:w970:dbl)
          n409 = Divide(x=w944, y=w943) -> (x/y=w941:dbl)
          n410 = Subtract(x=w947, y=w946) -> (x-y=w945:dbl)
          n411 = Increment(x=w970) -> (x+1=w965:dbl)
          n412 = case shown="True" "Hop Top" {
            tunnel: [w1059 w1063] -> w968
            tunnel: w965 -> [_ w1062]
            tunnel: w962 -> [_ w1060]
            frame False {
              n413 = local read "Hop Topography"() -> (w1059:dbl[][])
            }
            frame True {
              n414 = Initialize Array(0.0 ("disabled index (col)"), w1062, w1060) -> (w1063:dbl[][])
            }
          }
          n415 = Subtract(x=w940, y=w941) -> (x-y=w942:dbl)
          n416 = global read "Settings.vi" "Waypoints per hop"() -> (w954:dbl)
          n417 = Equal?(x=w954, y=3.0) -> (x = y?=w952:bool)
          n418 = Index Array "Real Z Position"(array=w975, index (row)=2 ("disabled index (row)"), index (col)=0 ("disabled index (col)")) -> (element=w951:dbl)
          n419 = case shown="True" w952 {
            tunnel: w968 -> [w981 w1032]
            tunnel: w951 -> [w982 w1031]
            tunnel: w967 -> [w991 w1030]
            tunnel: w965 -> [w990 w1028]
            tunnel: w961 -> [w984 w1027]
            tunnel: [w979 w1025] -> w950
            tunnel: w949 -> [w978 w1024]
            tunnel: w945 -> [w977 w1023]
            tunnel: w942 -> [w976 w1022]
            frame False {
              # "This is Y"
              # "This is N"
              # "Take every Nth line number starting from Y"
              n420 = global read "Settings.vi" "Waypoints per hop"() -> (w987:dbl)
              n421 = Equal?(x=w984, y=2.0) -> (x = y?=w983:bool)
              n422 = Quotient & Remainder(x=w984, y=w987) -> (x-y*floor(x/y)=w989:dbl)  [unwired: 1 out]
              n423 = case shown="True" w983 {
                tunnel: w982 -> [_ w995]
                tunnel: w981 -> [w992 w994]
                tunnel: [w992 w993] -> w980
                frame False {
                }
                frame True {
                  w996 = 0.0
                  n424 = Replace Array Subset(array=w994, new element=w995, index (row)=w996, index (col)=w996) -> (w993:dbl[][])
                }
              }
              n425 = Equal?(x=w989, y=5.0) -> (x = y?=w986:bool)
              n426 = case shown="True" w986 {
                tunnel: w990 -> [_ w1010]
                tunnel: w984 -> [_ w1012]
                tunnel: w982 -> [_ w1007]
                tunnel: w991 -> [_ w1006]
                tunnel: w980 -> [w997 w1002]
                tunnel: [w997 w1001] -> w979
                tunnel: w978 -> [_ w999]
                tunnel: w977 -> [_ w1000]
                tunnel: w976 -> [_ w998]
                frame False {
                }
                frame True {
                  # "Calculates x \nposition on graph"
                  # "Plot forward or backward?\n0,0,0,0,1,1,1,1,0,0,0,0"
                  # "Divide by number of pixels"
                  # "Calculates y line 0,0,0,0,1,1,1,1,2,2,2,2 etc"
                  # "Only one number per set of N\n1,2,3,4,5 etc"
                  n427 = global read "Settings.vi" "Waypoints per hop"() -> (w1005:dbl)
                  n428 = Quotient & Remainder(x=w1012, y=w1005) -> (floor(x/y)=w1004:dbl)  [unwired: 1 out]
                  n429 = Increment(x=w1004) -> (x+1=w1003:dbl)
                  n430 = Quotient & Remainder(x=w1003, y=w1010) -> (x-y*floor(x/y)=w1011:dbl, floor(x/y)=w1008:dbl)
                  n431 = Quotient & Remainder(x=w1008, y=2.0) -> (x-y*floor(x/y)=w1014:dbl)  [unwired: 1 out]
                  n432 = Equal To 0?(x=w1014) -> (x = 0?=w1013:bool)
                  n433 = case shown="False" w1013 {
                    tunnel: w1011 -> [w1017 w1021]
                    tunnel: [w1020 w1021] -> w1009
                    tunnel: w1010 -> [w1018 _]
                    frame False {
                      # "If not 0,\nPlot the reverse"
                      n434 = Decrement(x=w1018) -> (x-1=w1016:dbl)
                      n435 = Subtract(x=w1017, y=w1016) -> (x-y=w1019:dbl)
                      n436 = Absolute Value(x=w1019) -> (abs(x)=w1020:dbl)
                    }
                    frame True {
                    }
                  }
                  n437 = Replace Array Subset(array=w1002, new element=w1007, index (row)=w1009, index (col)=w1008) -> (w1001:dbl[][])
                  n438 = property class="IntGraph (strict)"(reference=w1006, "Value"=w1001, "XScale.Multiplier"=w999, "XScale.Offset"=w1000, "YScale.Multiplier"=w999, "YScale.Offset"=w998) -> ()  [unwired: 1 in, 2 out]
                }
              }
            }
            frame True {
              # "This is Y"
              # "This is N"
              # "Take every Nth line number starting from Y"
              n439 = global read "Settings.vi" "Waypoints per hop"() -> (w1026:dbl)
              n440 = Quotient & Remainder(x=w1027, y=w1026) -> (x-y*floor(x/y)=w1034:dbl)  [unwired: 1 out]
              n441 = Equal?(x=w1034, y=2.0) -> (x = y?=w1033:bool)
              n442 = case shown="False" w1033 {
                tunnel: w1028 -> [_ w1047]
                tunnel: w1027 -> [_ w1049]
                tunnel: w1032 -> [w1035 w1046]
                tunnel: w1031 -> [_ w1043]
                tunnel: w1030 -> [_ w1042]
                tunnel: [w1035 w1039] -> w1025
                tunnel: w1024 -> [_ w1036]
                tunnel: w1023 -> [_ w1038]
                tunnel: w1022 -> [_ w1037]
                frame False {
                }
                frame True {
                  # "Calculates x \nposition on graph"
                  # "Plot forward or backward?\n0,0,0,0,1,1,1,1,0,0,0,0"
                  # "Divide by number of pixels"
                  # "Calculates y line 0,0,0,0,1,1,1,1,2,2,2,2 etc"
                  # "Only one number per set of N\n1,2,3,4,5 etc"
                  n443 = global read "Settings.vi" "Waypoints per hop"() -> (w1041:dbl)
                  n444 = Quotient & Remainder(x=w1049, y=w1041) -> (floor(x/y)=w1040:dbl)  [unwired: 1 out]
                  n445 = Quotient & Remainder(x=w1040, y=w1047) -> (x-y*floor(x/y)=w1048:dbl, floor(x/y)=w1044:dbl)
                  n446 = Quotient & Remainder(x=w1044, y=2.0) -> (x-y*floor(x/y)=w1051:dbl)  [unwired: 1 out]
                  n447 = Equal To 0?(x=w1051) -> (x = 0?=w1050:bool)
                  n448 = case shown="False" w1050 {
                    tunnel: w1048 -> [w1054 w1058]
                    tunnel: [w1057 w1058] -> w1045
                    tunnel: w1047 -> [w1055 _]
                    frame False {
                      # "If not 0,\nPlot the reverse"
                      n449 = Decrement(x=w1055) -> (x-1=w1053:dbl)
                      n450 = Subtract(x=w1054, y=w1053) -> (x-y=w1056:dbl)
                      n451 = Absolute Value(x=w1056) -> (abs(x)=w1057:dbl)
                    }
                    frame True {
                    }
                  }
                  n452 = Replace Array Subset(array=w1046, new element=w1043, index (row)=w1045, index (col)=w1044) -> (w1039:dbl[][])
                  n453 = property class="IntGraph (strict)"(reference=w1042, "Value"=w1039, "XScale.Multiplier"=w1036, "XScale.Offset"=w1038, "YScale.Offset"=w1037, "YScale.Multiplier"=w1036) -> ()  [unwired: 1 in, 2 out]
                }
              }
            }
          }
          "Hop Topography" <- w950
        }
        frame True {
        }
      }
    }
    frame #26 {
      # "Hop\nX/Y/C1"
      n454 = Not A Number/Path/Refnum?(number/path/refnum=w1064) -> (NaN/Path/Refnum?=w1065:bool)
      n455 = case shown="False" w1065 {
        tunnel: w1066 -> [w1102 _]
        frame False {
          w1074 = 2.0 ("disabled index (col)")
          # "Y only goes up\n\nX goes back and forth"
          # "If new then set the array in the shape of the graph"
          # "New scan?"
          n456 = local read "Display Cluster"() -> (w1083:T1)
          n457 = Unbundle By Name(w1083) -> ("Hop X/Y/C1"=w1094:refnum<vi>, "X Width"=w1071:dbl, "Y Width"=w1070:dbl, "Hopping Distance"=w1078:dbl, "X Center"=w1072:dbl, "Y Center"=w1069:dbl)
          n458 = Index Array "LineNumber"(array=w1102, index (row)=9 ("disabled index (row)"), index (col)=0 ("disabled index (col)")) -> (element=w1089:dbl)
          n459 = Equal?(x=w1089, y=2.0) -> (x = y?=w1087:bool)
          n460 = Select(t=TRUE, s=w1087, f=FALSE) -> (s? t:f=w1084:bool)
          n461 = Divide(x=w1070, y=w1078) -> (x/y=w1091:dbl)
          n462 = Round Toward -Infinity(1:w1091) -> (0:w1092:dbl)
          n463 = Divide(x=w1071, y=w1078) -> (x/y=w1096:dbl)
          n464 = local write "Hop C1"(w1084) -> ()
          n465 = Increment(x=w1092) -> (x+1=w1090:dbl)
          n466 = Round Toward -Infinity(1:w1096) -> (0:w1097:dbl)
          n467 = Divide(x=w1071, y=w1074) -> (x/y=w1075:dbl)
          n468 = Increment(x=w1097) -> (x+1=w1093:dbl)
          n469 = case shown="False" "Hop C1" {
            tunnel: [w1186 w1190] -> w1095
            tunnel: w1093 -> [_ w1189]
            tunnel: w1090 -> [_ w1187]
            frame False {
              n470 = local read "Hop Current1"() -> (w1186:dbl[][])
            }
            frame True {
              n471 = Initialize Array(0.0 ("disabled index (col)"), w1189, w1187) -> (w1190:dbl[][])
            }
          }
          n472 = Divide(x=w1070, y=w1074) -> (x/y=w1073:dbl)
          n473 = Subtract(x=w1072, y=w1075) -> (x-y=w1068:dbl)
          n474 = Subtract(x=w1069, y=w1073) -> (x-y=w1067:dbl)
          n475 = global read "Settings.vi" "Waypoints per hop"() -> (w1082:dbl)
          n476 = Equal?(x=w1082, y=3.0) -> (x = y?=w1080:bool)
          n477 = Index Array "Current1"(array=w1102, index (row)=5 ("disabled index (row)"), index (col)=0 ("disabled index (col)")) -> (element=w1079:dbl)
          n478 = case shown="False" w1080 {
            tunnel: w1095 -> [w1108 w1159]
            tunnel: w1079 -> [w1109 w1158]
            tunnel: w1094 -> [w1118 w1157]
            tunnel: w1093 -> [w1117 w1155]
            tunnel: w1089 -> [w1111 w1154]
            tunnel: [w1106 w1152] -> w1076
            tunnel: w1078 -> [w1105 w1151]
            tunnel: w1068 -> [w1104 w1150]
            tunnel: w1067 -> [w1103 w1149]
            frame False {
              # "This is Y"
              # "This is N"
              # "Take every Nth line number starting from Y"
              n479 = global read "Settings.vi" "Waypoints per hop"() -> (w1114:dbl)
              n480 = Equal?(x=w1111, y=2.0) -> (x = y?=w1110:bool)
              n481 = Quotient & Remainder(x=w1111, y=w1114) -> (x-y*floor(x/y)=w1116:dbl)  [unwired: 1 out]
              n482 = case shown="True" w1110 {
                tunnel: w1109 -> [_ w1122]
                tunnel: w1108 -> [w1119 w1121]
                tunnel: [w1119 w1120] -> w1107
                frame False {
                }
                frame True {
                  w1123 = 0.0
                  n483 = Replace Array Subset(array=w1121, new element=w1122, index (row)=w1123, index (col)=w1123) -> (w1120:dbl[][])
                }
              }
              n484 = Equal?(x=w1116, y=5.0) -> (x = y?=w1113:bool)
              n485 = case shown="True" w1113 {
                tunnel: w1117 -> [_ w1137]
                tunnel: w1111 -> [_ w1139]
                tunnel: w1109 -> [_ w1134]
                tunnel: w1118 -> [_ w1133]
                tunnel: w1107 -> [w1124 w1129]
                tunnel: [w1124 w1128] -> w1106
                tunnel: w1105 -> [_ w1127]
                tunnel: w1104 -> [_ w1126]
                tunnel: w1103 -> [_ w1125]
                frame False {
                }
                frame True {
                  # "Calculates x \nposition on graph"
                  # "Plot forward or backward?\n0,0,0,0,1,1,1,1,0,0,0,0"
                  # "Divide by number of pixels"
                  # "Calculates y line 0,0,0,0,1,1,1,1,2,2,2,2 etc"
                  # "Only one number per set of N\n1,2,3,4,5 etc"
                  n486 = global read "Settings.vi" "Waypoints per hop"() -> (w1132:dbl)
                  n487 = Quotient & Remainder(x=w1139, y=w1132) -> (floor(x/y)=w1131:dbl)  [unwired: 1 out]
                  n488 = Increment(x=w1131) -> (x+1=w1130:dbl)
                  n489 = Quotient & Remainder(x=w1130, y=w1137) -> (x-y*floor(x/y)=w1138:dbl, floor(x/y)=w1135:dbl)
                  n490 = Quotient & Remainder(x=w1135, y=2.0) -> (x-y*floor(x/y)=w1141:dbl)  [unwired: 1 out]
                  n491 = Equal To 0?(x=w1141) -> (x = 0?=w1140:bool)
                  n492 = case shown="False" w1140 {
                    tunnel: w1138 -> [w1144 w1148]
                    tunnel: [w1147 w1148] -> w1136
                    tunnel: w1137 -> [w1145 _]
                    frame False {
                      # "If not 0,\nPlot the reverse"
                      n493 = Decrement(x=w1145) -> (x-1=w1143:dbl)
                      n494 = Subtract(x=w1144, y=w1143) -> (x-y=w1146:dbl)
                      n495 = Absolute Value(x=w1146) -> (abs(x)=w1147:dbl)
                    }
                    frame True {
                    }
                  }
                  n496 = Replace Array Subset(array=w1129, new element=w1134, index (row)=w1136, index (col)=w1135) -> (w1128:dbl[][])
                  n497 = property class="IntGraph (strict)"(reference=w1133, "Value"=w1128, "XScale.Multiplier"=w1127, "XScale.Offset"=w1126, "YScale.Offset"=w1125, "YScale.Multiplier"=w1127) -> ()  [unwired: 1 in, 2 out]
                }
              }
            }
            frame True {
              # "This is Y"
              # "This is N"
              # "Take every Nth line number starting from Y"
              n498 = global read "Settings.vi" "Waypoints per hop"() -> (w1153:dbl)
              n499 = Quotient & Remainder(x=w1154, y=w1153) -> (x-y*floor(x/y)=w1161:dbl)  [unwired: 1 out]
              n500 = Equal?(x=w1161, y=2.0) -> (x = y?=w1160:bool)
              n501 = case shown="True" w1160 {
                tunnel: w1155 -> [_ w1174]
                tunnel: w1154 -> [_ w1176]
                tunnel: w1159 -> [w1162 w1173]
                tunnel: w1158 -> [_ w1170]
                tunnel: w1157 -> [_ w1169]
                tunnel: [w1162 w1166] -> w1152
                tunnel: w1151 -> [_ w1163]
                tunnel: w1150 -> [_ w1165]
                tunnel: w1149 -> [_ w1164]
                frame False {
                }
                frame True {
                  # "Calculates x \nposition on graph"
                  # "Plot forward or backward?\n0,0,0,0,1,1,1,1,0,0,0,0"
                  # "Divide by number of pixels"
                  # "Calculates y line 0,0,0,0,1,1,1,1,2,2,2,2 etc"
                  # "Only one number per set of N\n1,2,3,4,5 etc"
                  n502 = global read "Settings.vi" "Waypoints per hop"() -> (w1168:dbl)
                  n503 = Quotient & Remainder(x=w1176, y=w1168) -> (floor(x/y)=w1167:dbl)  [unwired: 1 out]
                  n504 = Quotient & Remainder(x=w1167, y=w1174) -> (x-y*floor(x/y)=w1175:dbl, floor(x/y)=w1171:dbl)
                  n505 = Quotient & Remainder(x=w1171, y=2.0) -> (x-y*floor(x/y)=w1178:dbl)  [unwired: 1 out]
                  n506 = Equal To 0?(x=w1178) -> (x = 0?=w1177:bool)
                  n507 = case shown="False" w1177 {
                    tunnel: w1175 -> [w1181 w1185]
                    tunnel: [w1184 w1185] -> w1172
                    tunnel: w1174 -> [w1182 _]
                    frame False {
                      # "If not 0,\nPlot the reverse"
                      n508 = Decrement(x=w1182) -> (x-1=w1180:dbl)
                      n509 = Subtract(x=w1181, y=w1180) -> (x-y=w1183:dbl)
                      n510 = Absolute Value(x=w1183) -> (abs(x)=w1184:dbl)
                    }
                    frame True {
                    }
                  }
                  n511 = Replace Array Subset(array=w1173, new element=w1170, index (row)=w1172, index (col)=w1171) -> (w1166:dbl[][])
                  n512 = property class="IntGraph (strict)"(reference=w1169, "Value"=w1166, "XScale.Multiplier"=w1163, "XScale.Offset"=w1165, "YScale.Multiplier"=w1163, "YScale.Offset"=w1164) -> ()  [unwired: 1 in, 2 out]
                }
              }
            }
          }
          "Hop Current1" <- w1076
        }
        frame True {
        }
      }
    }
    frame #27 {
      # "Hop\nX/Y/C2"
      n513 = Not A Number/Path/Refnum?(number/path/refnum=w1191) -> (NaN/Path/Refnum?=w1192:bool)
      n514 = case shown="False" w1192 {
        tunnel: w1193 -> [w1229 _]
        frame False {
          w1201 = 2.0 ("disabled index (col)")
          # "Y only goes up\n\nX goes back and forth"
          # "If new then set the array in the shape of the graph"
          # "New scan?"
          n515 = local read "Display Cluster"() -> (w1210:T1)
          n516 = Unbundle By Name(w1210) -> ("Hop X/Y/C2"=w1221:refnum<vi>, "X Width"=w1199:dbl, "Y Width"=w1198:dbl, "Hopping Distance"=w1205:dbl, "X Center"=w1197:dbl, "Y Center"=w1196:dbl)
          n517 = Index Array "LineNumber"(array=w1229, index (row)=9 ("disabled index (row)"), index (col)=0 ("disabled index (col)")) -> (element=w1216:dbl)
          n518 = Equal?(x=w1216, y=2.0) -> (x = y?=w1214:bool)
          n519 = Select(t=TRUE, s=w1214, f=FALSE) -> (s? t:f=w1211:bool)
          n520 = Divide(x=w1198, y=w1205) -> (x/y=w1218:dbl)
          n521 = Round Toward -Infinity(1:w1218) -> (0:w1219:dbl)
          n522 = Divide(x=w1199, y=w1205) -> (x/y=w1223:dbl)
          n523 = local write "Hop C2"(w1211) -> ()
          n524 = Increment(x=w1219) -> (x+1=w1217:dbl)
          n525 = Round Toward -Infinity(1:w1223) -> (0:w1224:dbl)
          n526 = Increment(x=w1224) -> (x+1=w1220:dbl)
          n527 = case shown="False" "Hop C2" {
            tunnel: [w1313 w1317] -> w1222
            tunnel: w1220 -> [_ w1316]
            tunnel: w1217 -> [_ w1314]
            frame False {
              n528 = local read "Hop Current2"() -> (w1313:dbl[][])
            }
            frame True {
              n529 = Initialize Array(0.0 ("disabled index (col)"), w1316, w1314) -> (w1317:dbl[][])
            }
          }
          n530 = Divide(x=w1199, y=w1201) -> (x/y=w1202:dbl)
          n531 = Divide(x=w1198, y=w1201) -> (x/y=w1200:dbl)
          n532 = Subtract(x=w1197, y=w1202) -> (x-y=w1195:dbl)
          n533 = global read "Settings.vi" "Waypoints per hop"() -> (w1209:dbl)
          n534 = Subtract(x=w1196, y=w1200) -> (x-y=w1194:dbl)
          n535 = Equal?(x=w1209, y=3.0) -> (x = y?=w1207:bool)
          n536 = Index Array "Current2"(array=w1229, index (row)=6 ("disabled index (row)"), index (col)=0 ("disabled index (col)")) -> (element=w1206:dbl)
          n537 = case shown="False" w1207 {
            tunnel: w1222 -> [w1235 w1286]
            tunnel: w1206 -> [w1236 w1285]
            tunnel: w1221 -> [w1245 w1284]
            tunnel: w1220 -> [w1244 w1282]
            tunnel: w1216 -> [w1238 w1281]
            tunnel: [w1233 w1279] -> w1203
            tunnel: w1205 -> [w1230 w1278]
            tunnel: w1195 -> [w1231 w1277]
            tunnel: w1194 -> [w1232 w1276]
            frame False {
              # "This is Y"
              # "This is N"
              # "Take every Nth line number starting from Y"
              n538 = global read "Settings.vi" "Waypoints per hop"() -> (w1241:dbl)
              n539 = Equal?(x=w1238, y=2.0) -> (x = y?=w1237:bool)
              n540 = Quotient & Remainder(x=w1238, y=w1241) -> (x-y*floor(x/y)=w1243:dbl)  [unwired: 1 out]
              n541 = case shown="True" w1237 {
                tunnel: w1236 -> [_ w1249]
                tunnel: w1235 -> [w1246 w1248]
                tunnel: [w1246 w1247] -> w1234
                frame False {
                }
                frame True {
                  w1250 = 0.0
                  n542 = Replace Array Subset(array=w1248, new element=w1249, index (row)=w1250, index (col)=w1250) -> (w1247:dbl[][])
                }
              }
              n543 = Equal?(x=w1243, y=5.0) -> (x = y?=w1240:bool)
              n544 = case shown="True" w1240 {
                tunnel: w1244 -> [_ w1264]
                tunnel: w1238 -> [_ w1266]
                tunnel: w1236 -> [_ w1261]
                tunnel: w1245 -> [_ w1260]
                tunnel: w1234 -> [w1251 w1256]
                tunnel: [w1251 w1255] -> w1233
                tunnel: w1232 -> [_ w1254]
                tunnel: w1231 -> [_ w1253]
                tunnel: w1230 -> [_ w1252]
                frame False {
                }
                frame True {
                  # "Calculates x \nposition on graph"
                  # "Plot forward or backward?\n0,0,0,0,1,1,1,1,0,0,0,0"
                  # "Divide by number of pixels"
                  # "Calculates y line 0,0,0,0,1,1,1,1,2,2,2,2 etc"
                  # "Only one number per set of N\n1,2,3,4,5 etc"
                  n545 = global read "Settings.vi" "Waypoints per hop"() -> (w1259:dbl)
                  n546 = Quotient & Remainder(x=w1266, y=w1259) -> (floor(x/y)=w1258:dbl)  [unwired: 1 out]
                  n547 = Increment(x=w1258) -> (x+1=w1257:dbl)
                  n548 = Quotient & Remainder(x=w1257, y=w1264) -> (x-y*floor(x/y)=w1265:dbl, floor(x/y)=w1262:dbl)
                  n549 = Quotient & Remainder(x=w1262, y=2.0) -> (x-y*floor(x/y)=w1268:dbl)  [unwired: 1 out]
                  n550 = Equal To 0?(x=w1268) -> (x = 0?=w1267:bool)
                  n551 = case shown="False" w1267 {
                    tunnel: w1265 -> [w1271 w1275]
                    tunnel: [w1274 w1275] -> w1263
                    tunnel: w1264 -> [w1272 _]
                    frame False {
                      # "If not 0,\nPlot the reverse"
                      n552 = Decrement(x=w1272) -> (x-1=w1270:dbl)
                      n553 = Subtract(x=w1271, y=w1270) -> (x-y=w1273:dbl)
                      n554 = Absolute Value(x=w1273) -> (abs(x)=w1274:dbl)
                    }
                    frame True {
                    }
                  }
                  n555 = Replace Array Subset(array=w1256, new element=w1261, index (row)=w1263, index (col)=w1262) -> (w1255:dbl[][])
                  n556 = property class="IntGraph (strict)"(reference=w1260, "Value"=w1255, "XScale.Multiplier"=w1252, "XScale.Offset"=w1253, "YScale.Multiplier"=w1252, "YScale.Offset"=w1254) -> ()  [unwired: 1 in, 2 out]
                }
              }
            }
            frame True {
              # "This is Y"
              # "This is N"
              # "Take every Nth line number starting from Y"
              n557 = global read "Settings.vi" "Waypoints per hop"() -> (w1280:dbl)
              n558 = Quotient & Remainder(x=w1281, y=w1280) -> (x-y*floor(x/y)=w1288:dbl)  [unwired: 1 out]
              n559 = Equal?(x=w1288, y=2.0) -> (x = y?=w1287:bool)
              n560 = case shown="True" w1287 {
                tunnel: w1282 -> [_ w1301]
                tunnel: w1281 -> [_ w1303]
                tunnel: w1286 -> [w1289 w1300]
                tunnel: w1285 -> [_ w1297]
                tunnel: w1284 -> [_ w1296]
                tunnel: [w1289 w1293] -> w1279
                tunnel: w1278 -> [_ w1292]
                tunnel: w1277 -> [_ w1291]
                tunnel: w1276 -> [_ w1290]
                frame False {
                }
                frame True {
                  # "Calculates x \nposition on graph"
                  # "Plot forward or backward?\n0,0,0,0,1,1,1,1,0,0,0,0"
                  # "Divide by number of pixels"
                  # "Calculates y line 0,0,0,0,1,1,1,1,2,2,2,2 etc"
                  # "Only one number per set of N\n1,2,3,4,5 etc"
                  n561 = global read "Settings.vi" "Waypoints per hop"() -> (w1295:dbl)
                  n562 = Quotient & Remainder(x=w1303, y=w1295) -> (floor(x/y)=w1294:dbl)  [unwired: 1 out]
                  n563 = Quotient & Remainder(x=w1294, y=w1301) -> (x-y*floor(x/y)=w1302:dbl, floor(x/y)=w1298:dbl)
                  n564 = Quotient & Remainder(x=w1298, y=2.0) -> (x-y*floor(x/y)=w1305:dbl)  [unwired: 1 out]
                  n565 = Equal To 0?(x=w1305) -> (x = 0?=w1304:bool)
                  n566 = case shown="False" w1304 {
                    tunnel: w1302 -> [w1308 w1312]
                    tunnel: [w1311 w1312] -> w1299
                    tunnel: w1301 -> [w1309 _]
                    frame False {
                      # "If not 0,\nPlot the reverse"
                      n567 = Decrement(x=w1309) -> (x-1=w1307:dbl)
                      n568 = Subtract(x=w1308, y=w1307) -> (x-y=w1310:dbl)
                      n569 = Absolute Value(x=w1310) -> (abs(x)=w1311:dbl)
                    }
                    frame True {
                    }
                  }
                  n570 = Replace Array Subset(array=w1300, new element=w1297, index (row)=w1299, index (col)=w1298) -> (w1293:dbl[][])
                  n571 = property class="IntGraph (strict)"(reference=w1296, "Value"=w1293, "XScale.Multiplier"=w1292, "XScale.Offset"=w1291, "YScale.Multiplier"=w1292, "YScale.Offset"=w1290) -> ()  [unwired: 1 in, 2 out]
                }
              }
            }
          }
          "Hop Current2" <- w1203
        }
        frame True {
        }
      }
    }
    frame #28 {
      # "Hop\nX/Y/C3"
      n572 = Not A Number/Path/Refnum?(number/path/refnum=w1318) -> (NaN/Path/Refnum?=w1319:bool)
      n573 = case shown="False" w1319 {
        tunnel: w1320 -> [w1356 _]
        frame False {
          w1328 = 2.0 ("disabled index (col)")
          # "Y only goes up\n\nX goes back and forth"
          # "If new then set the array in the shape of the graph"
          # "New scan?"
          n574 = local read "Display Cluster"() -> (w1337:T1)
          n575 = Unbundle By Name(w1337) -> ("Hop X/Y/C3"=w1348:refnum<vi>, "X Width"=w1326:dbl, "Y Width"=w1325:dbl, "Hopping Distance"=w1332:dbl, "X Center"=w1324:dbl, "Y Center"=w1323:dbl)
          n576 = Index Array "LineNumber"(array=w1356, index (row)=9 ("disabled index (row)"), index (col)=0 ("disabled index (col)")) -> (element=w1343:dbl)
          n577 = Equal?(x=w1343, y=2.0) -> (x = y?=w1341:bool)
          n578 = Select(t=TRUE, s=w1341, f=FALSE) -> (s? t:f=w1338:bool)
          n579 = Divide(x=w1325, y=w1332) -> (x/y=w1345:dbl)
          n580 = Round Toward -Infinity(1:w1345) -> (0:w1346:dbl)
          n581 = Divide(x=w1326, y=w1332) -> (x/y=w1350:dbl)
          n582 = local write "Hop C3"(w1338) -> ()
          n583 = Increment(x=w1346) -> (x+1=w1344:dbl)
          n584 = Round Toward -Infinity(1:w1350) -> (0:w1351:dbl)
          n585 = Increment(x=w1351) -> (x+1=w1347:dbl)
          n586 = case shown="False" "Hop C3" {
            tunnel: [w1440 w1444] -> w1349
            tunnel: w1347 -> [_ w1443]
            tunnel: w1344 -> [_ w1441]
            frame False {
              n587 = local read "Hop Current3"() -> (w1440:dbl[][])
            }
            frame True {
              n588 = Initialize Array(0.0 ("disabled index (col)"), w1443, w1441) -> (w1444:dbl[][])
            }
          }
          n589 = Divide(x=w1326, y=w1328) -> (x/y=w1329:dbl)
          n590 = Divide(x=w1325, y=w1328) -> (x/y=w1327:dbl)
          n591 = global read "Settings.vi" "Waypoints per hop"() -> (w1336:dbl)
          n592 = Subtract(x=w1324, y=w1329) -> (x-y=w1322:dbl)
          n593 = Subtract(x=w1323, y=w1327) -> (x-y=w1321:dbl)
          n594 = Equal?(x=w1336, y=3.0) -> (x = y?=w1334:bool)
          n595 = Index Array "Current3"(array=w1356, index (row)=7 ("disabled index (row)"), index (col)=0 ("disabled index (col)")) -> (element=w1333:dbl)
          n596 = case shown="False" w1334 {
            tunnel: w1349 -> [w1362 w1413]
            tunnel: w1333 -> [w1363 w1412]
            tunnel: w1348 -> [w1372 w1411]
            tunnel: w1347 -> [w1371 w1409]
            tunnel: w1343 -> [w1365 w1408]
            tunnel: [w1360 w1406] -> w1330
            tunnel: w1332 -> [w1357 w1405]
            tunnel: w1322 -> [w1358 w1404]
            tunnel: w1321 -> [w1359 w1403]
            frame False {
              # "This is Y"
              # "This is N"
              # "Take every Nth line number starting from Y"
              n597 = global read "Settings.vi" "Waypoints per hop"() -> (w1368:dbl)
              n598 = Equal?(x=w1365, y=2.0) -> (x = y?=w1364:bool)
              n599 = Quotient & Remainder(x=w1365, y=w1368) -> (x-y*floor(x/y)=w1370:dbl)  [unwired: 1 out]
              n600 = case shown="True" w1364 {
                tunnel: w1363 -> [_ w1376]
                tunnel: w1362 -> [w1373 w1375]
                tunnel: [w1373 w1374] -> w1361
                frame False {
                }
                frame True {
                  w1377 = 0.0
                  n601 = Replace Array Subset(array=w1375, new element=w1376, index (row)=w1377, index (col)=w1377) -> (w1374:dbl[][])
                }
              }
              n602 = Equal?(x=w1370, y=5.0) -> (x = y?=w1367:bool)
              n603 = case shown="True" w1367 {
                tunnel: w1371 -> [_ w1391]
                tunnel: w1365 -> [_ w1393]
                tunnel: w1363 -> [_ w1388]
                tunnel: w1372 -> [_ w1387]
                tunnel: w1361 -> [w1378 w1383]
                tunnel: [w1378 w1382] -> w1360
                tunnel: w1359 -> [_ w1381]
                tunnel: w1358 -> [_ w1380]
                tunnel: w1357 -> [_ w1379]
                frame False {
                }
                frame True {
                  # "Calculates x \nposition on graph"
                  # "Plot forward or backward?\n0,0,0,0,1,1,1,1,0,0,0,0"
                  # "Divide by number of pixels"
                  # "Calculates y line 0,0,0,0,1,1,1,1,2,2,2,2 etc"
                  # "Only one number per set of N\n1,2,3,4,5 etc"
                  n604 = global read "Settings.vi" "Waypoints per hop"() -> (w1386:dbl)
                  n605 = Quotient & Remainder(x=w1393, y=w1386) -> (floor(x/y)=w1385:dbl)  [unwired: 1 out]
                  n606 = Increment(x=w1385) -> (x+1=w1384:dbl)
                  n607 = Quotient & Remainder(x=w1384, y=w1391) -> (x-y*floor(x/y)=w1392:dbl, floor(x/y)=w1389:dbl)
                  n608 = Quotient & Remainder(x=w1389, y=2.0) -> (x-y*floor(x/y)=w1395:dbl)  [unwired: 1 out]
                  n609 = Equal To 0?(x=w1395) -> (x = 0?=w1394:bool)
                  n610 = case shown="False" w1394 {
                    tunnel: w1392 -> [w1398 w1402]
                    tunnel: [w1401 w1402] -> w1390
                    tunnel: w1391 -> [w1399 _]
                    frame False {
                      # "If not 0,\nPlot the reverse"
                      n611 = Decrement(x=w1399) -> (x-1=w1397:dbl)
                      n612 = Subtract(x=w1398, y=w1397) -> (x-y=w1400:dbl)
                      n613 = Absolute Value(x=w1400) -> (abs(x)=w1401:dbl)
                    }
                    frame True {
                    }
                  }
                  n614 = Replace Array Subset(array=w1383, new element=w1388, index (row)=w1390, index (col)=w1389) -> (w1382:dbl[][])
                  n615 = property class="IntGraph (strict)"(reference=w1387, "Value"=w1382, "XScale.Multiplier"=w1379, "XScale.Offset"=w1380, "YScale.Multiplier"=w1379, "YScale.Offset"=w1381) -> ()  [unwired: 1 in, 2 out]
                }
              }
            }
            frame True {
              # "This is Y"
              # "This is N"
              # "Take every Nth line number starting from Y"
              n616 = global read "Settings.vi" "Waypoints per hop"() -> (w1407:dbl)
              n617 = Quotient & Remainder(x=w1408, y=w1407) -> (x-y*floor(x/y)=w1415:dbl)  [unwired: 1 out]
              n618 = Equal?(x=w1415, y=2.0) -> (x = y?=w1414:bool)
              n619 = case shown="True" w1414 {
                tunnel: w1409 -> [_ w1428]
                tunnel: w1408 -> [_ w1430]
                tunnel: w1413 -> [w1416 w1427]
                tunnel: w1412 -> [_ w1424]
                tunnel: w1411 -> [_ w1423]
                tunnel: [w1416 w1420] -> w1406
                tunnel: w1405 -> [_ w1417]
                tunnel: w1404 -> [_ w1419]
                tunnel: w1403 -> [_ w1418]
                frame False {
                }
                frame True {
                  # "Calculates x \nposition on graph"
                  # "Plot forward or backward?\n0,0,0,0,1,1,1,1,0,0,0,0"
                  # "Divide by number of pixels"
                  # "Calculates y line 0,0,0,0,1,1,1,1,2,2,2,2 etc"
                  # "Only one number per set of N\n1,2,3,4,5 etc"
                  n620 = global read "Settings.vi" "Waypoints per hop"() -> (w1422:dbl)
                  n621 = Quotient & Remainder(x=w1430, y=w1422) -> (floor(x/y)=w1421:dbl)  [unwired: 1 out]
                  n622 = Quotient & Remainder(x=w1421, y=w1428) -> (x-y*floor(x/y)=w1429:dbl, floor(x/y)=w1425:dbl)
                  n623 = Quotient & Remainder(x=w1425, y=2.0) -> (x-y*floor(x/y)=w1432:dbl)  [unwired: 1 out]
                  n624 = Equal To 0?(x=w1432) -> (x = 0?=w1431:bool)
                  n625 = case shown="False" w1431 {
                    tunnel: w1429 -> [w1435 w1439]
                    tunnel: [w1438 w1439] -> w1426
                    tunnel: w1428 -> [w1436 _]
                    frame False {
                      # "If not 0,\nPlot the reverse"
                      n626 = Decrement(x=w1436) -> (x-1=w1434:dbl)
                      n627 = Subtract(x=w1435, y=w1434) -> (x-y=w1437:dbl)
                      n628 = Absolute Value(x=w1437) -> (abs(x)=w1438:dbl)
                    }
                    frame True {
                    }
                  }
                  n629 = Replace Array Subset(array=w1427, new element=w1424, index (row)=w1426, index (col)=w1425) -> (w1420:dbl[][])
                  n630 = property class="IntGraph (strict)"(reference=w1423, "Value"=w1420, "XScale.Multiplier"=w1417, "XScale.Offset"=w1419, "YScale.Multiplier"=w1417, "YScale.Offset"=w1418) -> ()  [unwired: 1 in, 2 out]
                }
              }
            }
          }
          "Hop Current3" <- w1330
        }
        frame True {
        }
      }
    }
    frame #29 {
      # "V vs Phase"
      n631 = Not A Number/Path/Refnum?(number/path/refnum=w1447) -> (NaN/Path/Refnum?=w1448:bool)
      n632 = case shown="False" w1448 {
        tunnel: w1447 -> [w1453 _]
        tunnel: w1445 -> [w1452 _]
        tunnel: w1446 -> [w1451 _]
        frame False {
          n633 = Index Array ("Oscillation Amplitude")(array=w1452, index (row)=3 ("disabled index (row)"), index (col)=0) -> (element=w1456:dbl)
          n634 = Index Array ("Oscillation Amplitude")(array=w1452, index (row)=11 ("disabled index (row)"), index (col)=0) -> (element=w1454:dbl)
          n635 = call "XY Chart Buffer_PINK.vi"("clear first (no:F)"=w1451, "chart length (points)"=10000, "YNew"=w1454, "XNew"=w1456) -> ("Value Y"=w1464:dbl[], "Value X"=w1463:dbl[])  [unwired: 6 in]
          n636 = Bundle("Value X"=w1463, "Value Y"=w1464) -> (w1462:cluster{"Value X":dbl[], "Value Y":dbl[]})  [unwired: 1 in]
          n637 = Build Array(w1462) -> (w1457:cluster{"Value X":dbl[], "Value Y":dbl[]}[])
          n638 = property class="XYGraph (strict)"(reference=w1453, "Value"=w1457, "XScale.NameLbl.Text"="Potential (V)" ("X Scale.Name Label.Text"), "YScale.NameLbl.Text"="Phase (deg)" ("Y Scale.Name Label.Text")) -> ()  [unwired: 1 in, 2 out]
        }
        frame True {
        }
      }
    }
    frame #30 {
      # "V2 vs C1"
      n639 = Not A Number/Path/Refnum?(number/path/refnum=w1465) -> (NaN/Path/Refnum?=w1468:bool)
      n640 = case shown="False" w1468 {
        tunnel: w1465 -> [w1474 _]
        tunnel: w1466 -> [w1473 _]
        tunnel: w1467 -> [w1472 _]
        frame False {
          n641 = Index Array ("Oscillation Amplitude")(array=w1473, index (row)=4 ("disabled index (row)"), index (col)=0) -> (element=w1477:dbl)
          n642 = Index Array ("Oscillation Amplitude")(array=w1473, index (row)=5 ("disabled index (row)"), index (col)=0) -> (element=w1475:dbl)
          n643 = call "XY Chart Buffer_PINK.vi"("clear first (no:F)"=w1472, "chart length (points)"=10000, "YNew"=w1475, "XNew"=w1477) -> ("Value Y"=w1485:dbl[], "Value X"=w1484:dbl[])  [unwired: 6 in]
          n644 = Bundle("Value X"=w1484, "Value Y"=w1485) -> (w1483:cluster{"Value X":dbl[], "Value Y":dbl[]})  [unwired: 1 in]
          n645 = Build Array(w1483) -> (w1478:cluster{"Value X":dbl[], "Value Y":dbl[]}[])
          n646 = property class="XYGraph (strict)"(reference=w1474, "Value"=w1478, "XScale.NameLbl.Text"="Potential (V2)" ("X Scale.Name Label.Text"), "YScale.NameLbl.Text"="Current 1 (nA)" ("Y Scale.Name Label.Text"), "YScale.Multiplier"=1000000000.0 ("Y Scale.Offset and Multiplier:Multiplier")) -> ()  [unwired: 1 in, 2 out]
        }
        frame True {
        }
      }
    }
    frame #31 {
      # "V2 vs C2"
      n647 = Not A Number/Path/Refnum?(number/path/refnum=w1486) -> (NaN/Path/Refnum?=w1489:bool)
      n648 = case shown="False" w1489 {
        tunnel: w1486 -> [w1495 _]
        tunnel: w1487 -> [w1494 _]
        tunnel: w1488 -> [w1493 _]
        frame False {
          n649 = Index Array ("Oscillation Amplitude")(array=w1494, index (row)=4 ("disabled index (row)"), index (col)=0) -> (element=w1498:dbl)
          n650 = Index Array ("Oscillation Amplitude")(array=w1494, index (row)=6 ("disabled index (row)"), index (col)=0) -> (element=w1496:dbl)
          n651 = call "XY Chart Buffer_PINK.vi"("clear first (no:F)"=w1493, "chart length (points)"=10000, "YNew"=w1496, "XNew"=w1498) -> ("Value Y"=w1506:dbl[], "Value X"=w1505:dbl[])  [unwired: 6 in]
          n652 = Bundle("Value X"=w1505, "Value Y"=w1506) -> (w1504:cluster{"Value X":dbl[], "Value Y":dbl[]})  [unwired: 1 in]
          n653 = Build Array(w1504) -> (w1499:cluster{"Value X":dbl[], "Value Y":dbl[]}[])
          n654 = property class="XYGraph (strict)"(reference=w1495, "Value"=w1499, "XScale.NameLbl.Text"="Potential (V2)" ("X Scale.Name Label.Text"), "YScale.NameLbl.Text"="Current 2 (nA)" ("Y Scale.Name Label.Text"), "YScale.Multiplier"=1000000000.0 ("Y Scale.Offset and Multiplier:Multiplier")) -> ()  [unwired: 1 in, 2 out]
        }
        frame True {
        }
      }
    }
    frame #32 {
      # "V2 vs C3"
      n655 = Not A Number/Path/Refnum?(number/path/refnum=w1507) -> (NaN/Path/Refnum?=w1510:bool)
      n656 = case shown="False" w1510 {
        tunnel: w1507 -> [w1516 _]
        tunnel: w1508 -> [w1515 _]
        tunnel: w1509 -> [w1514 _]
        frame False {
          n657 = Index Array ("Oscillation Amplitude")(array=w1515, index (row)=4 ("disabled index (row)"), index (col)=0) -> (element=w1519:dbl)
          n658 = Index Array ("Oscillation Amplitude")(array=w1515, index (row)=7 ("disabled index (row)"), index (col)=0) -> (element=w1517:dbl)
          n659 = call "XY Chart Buffer_PINK.vi"("clear first (no:F)"=w1514, "chart length (points)"=10000, "YNew"=w1517, "XNew"=w1519) -> ("Value Y"=w1527:dbl[], "Value X"=w1526:dbl[])  [unwired: 6 in]
          n660 = Bundle("Value X"=w1526, "Value Y"=w1527) -> (w1525:cluster{"Value X":dbl[], "Value Y":dbl[]})  [unwired: 1 in]
          n661 = Build Array(w1525) -> (w1520:cluster{"Value X":dbl[], "Value Y":dbl[]}[])
          n662 = property class="XYGraph (strict)"(reference=w1516, "Value"=w1520, "XScale.NameLbl.Text"="Potential (V2)" ("X Scale.Name Label.Text"), "YScale.NameLbl.Text"="Current 3 (nA)" ("Y Scale.Name Label.Text"), "YScale.Multiplier"=1000000000.0 ("Y Scale.Offset and Multiplier:Multiplier")) -> ()  [unwired: 1 in, 2 out]
        }
        frame True {
        }
      }
    }
  }
